vi "Main.vi"(11 "Module Admin":refnum<class "Delacor_lib_QMH_Module Admin.lvclass">) -> ()   [LabVIEW 2025, in "Scripting Server.lvlib"]
doc: "This template is based off of the Queued Message Handler design pattern and the Queued Message Handler project template that ships with LabVIEW.\n\nThe main difference is that the queue is private to this module and communication between modules is performed via Broadcast and Request events.\n\nRequest events are wrapped in public API methods and are handled in the Event Handling Loop (EHL) of this VI. Any module can register for Broadcast events sent by this module. The EHL generates messages based on user interface actions.\n\nThe Message Handling Loop (MHL) processes messages generated by the EHL, or by other messages. The messages are string values, so new messages can be added easily to the Message Cases case structure in the MHL. Each message cluster can also provide an optional value for Message Data, which is a variant that can be converted to whatever message-specific data is required.\n_____\nBased on DQMH Dev Tools: Project Template 7.1.0.1503."
uses:
  Scripting Server.lvlib
  <vilib>/Delacor/Delacor QMH/Libraries/Message Queue_class/Delacor_lib_QMH_Message Queue.lvclass/Delacor_lib_QMH_Message Queue.ctl
  <vilib>/Delacor/Delacor QMH/Libraries/Module Admin_class/Delacor_lib_QMH_Module Admin.lvclass/Delacor_lib_QMH_Module Admin.ctl
  <vilib>/Delacor/Delacor QMH/Libraries/Message Queue_class/Delacor_lib_QMH_Message Queue.lvclass
  Module Data--cluster.ctl
  <vilib>/Utility/miscctls.llb/LVPointTypeDef.ctl
  <vilib>/Delacor/Delacor QMH/Libraries/Message Queue_class/Delacor_lib_QMH_Enqueue Message (Single).vi
  Stop Argument--cluster.ctl
  <vilib>/Delacor/Delacor QMH/Libraries/Module Admin_class/Delacor_lib_QMH_Module Admin.lvclass
  New VI (Reply Payload)--cluster.ctl
  New VI Argument--cluster.ctl
  Add Object Argument--cluster.ctl
  Add Object (Reply Payload)--cluster.ctl
  Connect Objects (Reply Payload)--cluster.ctl
  Connect Objects Argument--cluster.ctl
  Get Object Terminals (Reply Payload)--cluster.ctl
  Get Object Terminals Argument--cluster.ctl
  get vi error list (Reply Payload)--cluster.ctl
  get vi error list Argument--cluster.ctl
  Cleanup VI (Reply Payload)--cluster.ctl
  Cleanup VI Argument--cluster.ctl
  create_control (Reply Payload)--cluster.ctl
  create_control Argument--cluster.ctl
  Run VI (Reply Payload)--cluster.ctl
  Run VI Argument--cluster.ctl
  add_to_selection (Reply Payload)--cluster.ctl
  add_to_selection Argument--cluster.ctl
  clear_selection_list (Reply Payload)--cluster.ctl
  clear_selection_list Argument--cluster.ctl
  remove_from_selection (Reply Payload)--cluster.ctl
  remove_from_selection Argument--cluster.ctl
  enclose_selection (Reply Payload)--cluster.ctl
  enclose_selection Argument--cluster.ctl
  rename_object (Reply Payload)--cluster.ctl
  rename_object Argument--cluster.ctl
  set_value (Reply Payload)--cluster.ctl
  set_value Argument--cluster.ctl
  delete_object (Reply Payload)--cluster.ctl
  delete_object Argument--cluster.ctl
  save_vi (Reply Payload)--cluster.ctl
  save_vi Argument--cluster.ctl
  get_structure_diagram (Reply Payload)--cluster.ctl
  get_structure_diagram Argument--cluster.ctl
  add_subvi (Reply Payload)--cluster.ctl
  add_subvi Argument--cluster.ctl
  connect_to_pane (Reply Payload)--cluster.ctl
  connect_to_pane Argument--cluster.ctl
  get_object_help (Reply Payload)--cluster.ctl
  get_object_help Argument--cluster.ctl
  get_loop_conditional_terminal (Reply Payload)--cluster.ctl
  get_loop_conditional_terminal Argument--cluster.ctl
  show_conditional_terminal (Reply Payload)--cluster.ctl
  show_conditional_terminal Argument--cluster.ctl
  get_loop_iteration_terminal (Reply Payload)--cluster.ctl
  get_loop_iteration_terminal Argument--cluster.ctl
  Config Data.ctl
  Read Config Data Argument--cluster.ctl
  get_allowed_paths (Reply Payload)--cluster.ctl
  get_allowed_paths Argument--cluster.ctl
  create_project (Reply Payload)--cluster.ctl
  create_project Argument--cluster.ctl
  Set Allowed Paths Argument--cluster.ctl
  open_vi (Reply Payload)--cluster.ctl
  open_vi Argument--cluster.ctl
panel:
  in  "Ring 2":i32(ring)=2125 items=[".NET Container"=2125, ".NET Refnum"=3441, "2D Picture"=3508, "3D Picture"=23776, "Absolute Value"=1054, "Accept TLS"=1732, "Access Rights"=1412, "ActiveX Container"=2072, "Add"=1050, "Add (with error terminals)"=3915, "Add Array Elements"=1903, "Add Entropy"=1738, "Add Private Key To TLS Configuration"=1735, "Add Trusted Certificate To TLS Configuration"=1736, "Agitator"=3831, "AllSpoll"=1960, "Always Copy"=2400, "And"=1061, "And Array Elements"=1911, "Append True/False String"=1511, "Application Refnum"=3412, "Array (block diagram constant)"=2070, "Array (classic)"=3300, "Array (modern)"=21608, "Array Interface Control"=23777, "Array Max & Min"=1907, "Array of Strings to Path"=1422, "Array Size"=1809, "Array Subset"=2044, "Array To Cluster"=1168, "Array To Spreadsheet String"=1540, "ArrayMemInfo"=2412, "Assert Structural Type Match"=2416, "Assert Structural Type Mismatch"=2464, "Atmospheric Tank (classic)"=3070, "Atmospheric Tank (modern)"=21751, "Automation Close"=8001, "Automation Open"=8000, "Automation Refnum"=3410, "Avogadro Constant (1/mol)"=23520, "Base 10 Logarithm Of e"=23512, "Bin #1"=3073, "Bin #2"=21755, "Bitpack to Array"=3135, "Bluetooth Close Connection"=9148, "Bluetooth Create Listener"=9151, "Bluetooth Discover"=9152, "Bluetooth Network Connection Refnum"=3468, "Bluetooth Open Connection"=9153, "Bluetooth Read"=9149, "Bluetooth Wait On Listener"=9147, "Bluetooth Write"=9150, "Boolean Array To Number"=1815, "Boolean To (0,1)"=1167, "Build Array"=2041, "Build Cluster Array"=2047, "Build Map"=2463, "Build Matrix"=8500, "Build Path"=1419, "Build Set"=2462, "Build Waveform"=2066, "Bundle"=2049, "Bundle By Name"=2057, "Byte Array To String"=1609, "Byte Array To UTF-8 String"=1651, "Byte Stream File Refnum"=3408, "Call By Reference"=3901, "Call Chain"=1999, "Call Library Function Node"=2062, "Call MATLAB Function"=24210, "Call Parent Class Method"=2354, "CAN Channel (block diagram constant)"=2124, "CAN Channel (classic)"=3340, "CAN Channel (modern)"=21817, "CAN Channel (system)"=21966, "CAN Interface (block diagram constant)"=2123, "CAN Interface (classic)"=3339, "CAN Interface (modern)"=21815, "CAN Interface (system)"=21964, "CAN Task (block diagram constant)"=3471, "CAN Task (classic)"=3470, "CAN Task (modern)"=21789, "CAN Task (system)"=21963, "Cancel Button (modern)"=21739, "Cancel Button (system)"=3131, "Cancel Notification"=9107, "Carriage Return Constant"=23500, "Case Structure"=2001, "Cast Unit Bases"=1079, "Check Valve"=3833, "Checkbox (classic)"=3117, "CheckBox (modern)"=21924, "Checkbox (system)"=3132, "Class Specifier Constant"=2094, "Classic Color Box"=3013, "Classic Color Ramp"=3022, "Classic Horizontal Slide Switch"=3114, "Classic Vertical Slide"=3004, "Clear Fixed-Point Overflow Status"=5562, "Close File"=8052, "Close File (deprecated)"=1405, "Close MATLAB Session"=24209, "Close Python Session"=24207, "Close Reference"=8011, "Close TLS Configuration"=1741, "Close Variable Connection"=23783, "Closure Structure"=2372, "Cluster (classic)"=3400, "Cluster (modern)"=21607, "Cluster Constant"=2071, "Cluster To Array"=1169, "Code Interface Node"=2050, "Coerce To Type"=2402, "Collection Size"=2450, "Color Box Constant"=2120, "Color Box Thin Border"=2905, "Colored Rectangle (broken?)"=3625, "Combo Box (classic)"=3304, "Combo Box (modern)"=21604, "Combo Box (system)"=21917, "Combo Box Constant"=2088, "Complex Conjugate"=1048, "Complex To Polar"=1045, "Complex To Re/Im"=1044, "Compound Arithmetic"=2200, "Compressor"=3832, "Concatenate Strings"=2040, "Conditional Disable Structure"=2064, "Constructor Node"=3904, "Control & Simulation Loop"=2099, "Control Help Window"=1353, "Control Online Help"=1355, "Control Refnum"=3419, "Convert Unit"=2059, "Conveyer"=3827, "Copy"=8053, "Copy (deprecated)"=1416, "Cosecant"=1204, "Cosine"=1201, "Cotangent"=1205, "CPU Information"=24130, "Create Folder"=8055, "Create Network Stream Endpoint"=23793, "Create Network Stream Reader Endpoint"=23811, "Create Network Stream Writer Endpoint"=23810, "Create Stream"=23796, "Create Unique Network Stream Endpoint"=23795, "Create Unique Network Stream Reader Endpoint"=23807, "Create Unique Network Stream Writer Endpoint"=23806, "Create User Event"=2073, "Current Processor ID"=24131, "Current VI's Menubar"=9000, "Current VI's Path"=1426, "DAQmx Analog Trigger Source (block diagram constant)"=2119, "DAQmx Analog Trigger Source (classic)"=3336, "DAQmx Analog Trigger Source (modern)"=21774, "DAQmx Analog Trigger Source (system)"=21951, "DAQmx Device Name (block diagram constant)"=2093, "DAQmx Device Name (classic)"=3318, "DAQmx Device Name (modern)"=21773, "DAQmx Device Name (system)"=21950, "DAQmx Global Channel (block diagram constant)"=3430, "DAQmx Global Channel (classic)"=3443, "DAQmx Global Channel (modern)"=21770, "DAQmx Global Channel (system)"=21957, "DAQmx Physical Channel (block diagram constant)"=2118, "DAQmx Physical Channel (classic)"=3335, "DAQmx Physical Channel (modern)"=21777, "DAQmx Physical Channel (system)"=21954, "DAQmx Scale Name (block diagram constant)"=2116, "DAQmx Scale Name (classic)"=3317, "DAQmx Scale Name (modern)"=21775, "DAQmx Scale Name (system)"=21952, "DAQmx Switch (block diagram constant)"=2121, "DAQmx Switch (classic)"=3337, "DAQmx Switch (modern)"=21776, "DAQmx Switch (system)"=21953, "DAQmx Task Name (block diagram constant)"=3434, "DAQmx Task Name (classic)"=3442, "DAQmx Task Name (modern)"=21778, "DAQmx Task Name (system)"=21959, "DAQmx Terminal (block diagram constant)"=2117, "DAQmx Terminal (classic)"=3319, "DAQmx Terminal (modern)"=21781, "DAQmx Terminal (system)"=21955, "Data Cache Size"=24132, "Data Log File Refnum"=3402, "Data Value Reference"=3476, "Data Value Reference Constant"=24134, "DataSocket Close"=1085, "DataSocket Open"=1084, "DataSocket Read"=1086, "DataSocket Refnum"=3417, "DataSocket Write"=1087, "Date/Time To Seconds"=1308, "Decimal Digit?"=1119, "Decimal String To Number"=1184, "Decimate 1D Array"=2046, "DecomposeLockDataValRef"=2406, "DecomposeVariant"=2404, "Decrement"=1058, "Default Directory"=1427, "Delete"=8056, "Delete (deprecated)"=1417, "Delete Data Value Reference"=2409, "Delete From Array"=3912, "Delete Menu Items"=9004, "Delete Variant Attribute"=8206, "Delete Waveform Attribute"=8209, "Deny Access"=8057, "Dequeue Element"=9113, "Destroy Stream Endpoint"=23794, "Destroy User Event"=2075, "DevClear"=1961, "DevClearList"=1962, "Device Control/Status"=1433, "Device Refnum"=3405, "Diagram Disable Structure"=2054, "Dial (classic)"=3050, "Dial (modern)"=21732, "Digital Data (classic)"=3210, "Digital Data (modern)"=21216, "Digital Waveform Graph (classic)"=3511, "Digital Waveform Graph (modern)"=21718, "Direct Variable Read"=23785, "Direct Variable Write"=23788, "Divide"=1053, "Divide (with error terminals)"=3918, "Dlg Horiz Scrollbar"=21905, "Dlg Mac Group Box"=32514, "Dlg Numeric #1"=2100, "Dlg Numeric #2"=3006, "Dlg String"=2110, "Dlg Vert Scrollbar"=21906, "Down Arrow"=3824, "Down Bow Valve (flat)"=3707, "Down Bow Valve (outline)"=3807, "Down Bow Valve (shaded)"=21767, "Down Rect Valve (flat)"=3706, "Down Rect Valve (outline)"=3806, "Down Rect Valve (shaded)"=21766, "Down Tee (flat)"=3818, "Down Tee (shaded)"=3718, "Dynamic FPGA Interface Cast"=5690, "Eased Corner Rectangle"=32513, "Element of Set?"=2454, "Elementary Charge (C)"=23517, "Empty Array?"=23063, "Empty Collection?"=2451, "Empty Path Constant"=23523, "Empty String Constant"=23503, "Empty String/Path?"=1112, "Enable Menu Tracking"=9002, "EnableLocal"=1963, "EnableRemote"=1964, "End of Line Constant"=23525, "Enqueue Element"=9111, "Enqueue Element At Opposite End"=9129, "Enum (classic)"=3023, "Enum (modern)"=21605, "Enum (system)"=3062, "Enum Constant"=2090, "EOF"=1410, "Equal To 0?"=1113, "Equal?"=1102, "Error Ring Constant"=2039, "Event Callback Refnum"=3435, "Event Data Node"=2102, "Event Structure"=2052, "Exchanger"=3828, "Exclusive Or"=1063, "Exponential"=1211, "Exponential (Arg) -1"=1222, "Expression Node"=2201, "False Constant"=2006, "Feedback Node"=2353, "FieldPoint IO Point (block diagram constant)"=3440, "FieldPoint IO Point (classic)"=3439, "FieldPoint IO Point (modern)"=21784, "FIFO Refnum"=3474, "File Dialog"=8058, "File Dialog (deprecated)"=8081, "File Path Control (classic)"=3203, "File Path Control (modern)"=21730, "File Path Control (system)"=21922, "File Path Indicator (classic)"=3204, "File Path Indicator (modern)"=21731, "File/Directory Info"=8082, "File/Directory Info (deprecated)"=1413, "FindLstn"=1965, "FindRQS"=1966, "First Call?"=1083, "Fixed-Point Overflow?"=5565, "Fixed-Point to Integer Cast"=5566, "Flat Box"=3602, "Flat Circle"=3605, "Flat Down Triangle"=3623, "Flat Frame"=3608, "Flat Left Triangle"=3620, "Flat Right Triangle"=3621, "Flat Round Button"=3102, "Flat Rounded Box"=3611, "Flat Sequence Structure"=2069, "Flat Square Button"=3103, "Flat Up Triangle"=3622, "Flatten To JSON"=24201, "Flatten To String"=1164, "Flatten To XML"=8402, "Flattened String To Variant"=8202, "Floating Point Equal?"=23064, "Flush Event Queue"=2135, "Flush File"=8059, "Flush File (deprecated)"=1406, "Flush Queue"=9114, "Flush Stream"=23808, "For Loop"=2002, "Fork"=2194, "Format Date/Time String"=8100, "Format Into File"=2083, "Format Into String"=2081, "Format Value"=1512, "Formula Node"=2004, "FPGA Refnum to Session"=2322, "Fract/Exp String To Number"=1187, "Framed Color Box (classic)"=3008, "Framed Color Box (modern)"=21019, "Free Label"=2321, "Furnace"=3829, "Gauge (classic)"=3040, "Gauge (modern)"=21009, "Gauge for Simon"=32600, "Generate Front Panel Activity"=1329, "Generate Occurrence"=1700, "Generate User Event"=2074, "Generate User-Defined Trace Event"=2250, "Get Control Values by Index"=24204, "Get Datalog Position"=8061, "Get Date/Time In Seconds"=1303, "Get Date/Time String"=1600, "Get Drag Drop Data"=9154, "Get File Position"=8062, "Get File Size"=8063, "Get Fixed-Point Components"=11163, "Get Help Window Status"=1354, "Get Matrix Diagonal"=8501, "Get Matrix Elements"=8502, "Get Menu Item Info"=9005, "Get Menu Selection"=9001, "Get Menu Short Cut Info"=9007, "Get Notifier Status"=9103, "Get Number of Records"=8064, "Get Permissions"=8065, "Get Queue Status"=9110, "Get Submatrix"=8503, "Get Type and Creator"=8066, "Get Variant Attribute"=8205, "Get Volume Info"=8067, "Get Waveform Attribute"=8208, "Get Waveform Components"=2067, "Global Variable"=2060, "GPIB Clear"=1954, "GPIB Initialization"=1957, "GPIB Misc"=1956, "GPIB Read"=1951, "GPIB Serial Poll"=1955, "GPIB Status"=1959, "GPIB Trigger"=1953, "GPIB Wait"=1958, "GPIB Write"=1950, "Gravitational Constant (N m2/kg2)"=23519, "Greater Or Equal To 0?"=1114, "Greater Or Equal?"=1103, "Greater Than 0?"=1117, "Greater?"=1110, "Handle Peek"=1604, "Handle Poke"=1605, "Hex Digit?"=1123, "Hexadecimal String To Number"=1185, "Hopper #1"=21754, "Hopper #2"=3072, "Horiz Line"=3821, "Horiz Pipe (flat)"=3810, "Horiz Pipe (shaded)"=3710, "Horizontal Button Box"=3636, "Horizontal Fill Slide (classic)"=3012, "Horizontal Fill Slide (modern)"=21100, "Horizontal Gradient Oval"=32502, "Horizontal Gradient Rectangle"=32504, "Horizontal Gradient Rounded Rectangle"=32507, "Horizontal Graduated Bar"=21106, "Horizontal Pointer Slide (classic)"=3011, "Horizontal Pointer Slide (modern)"=21101, "Horizontal Pointer Slide (system)"=21902, "Horizontal Progress Bar (modern)"=21102, "Horizontal Progress Bar (system)"=21910, "Horizontal Scrollbar"=21110, "Horizontal Slide (classic)"=3010, "Horizontal Slide (system)"=21904, "Horizontal Smooth Box"=3633, "Horizontal Splitter Bar"=21861, "Horizontal Splitter Bar (Classic)"=21863, "Horizontal Splitter Bar (NXG Style)"=21867, "Horizontal Splitter Bar (System)"=21865, "Horizontal Switch"=3108, "Horizontal Tank"=3071, "Horizontal Toggle Switch (classic)"=3110, "Horizontal Toggle Switch (modern)"=21700, "Hyperbolic Cosecant"=23053, "Hyperbolic Cosine"=1215, "Hyperbolic Cotangent"=23055, "Hyperbolic Secant"=23054, "Hyperbolic Sine"=1214, "Hyperbolic Tangent"=1216, "IMAQ Session"=3415, "Implies"=1080, "In Place Element Structure"=2360, "In Range and Coerce"=1127, "Include Fixed-Point Overflow Status"=5564, "Increment"=1057, "Index & Bundle Cluster Array"=2056, "Index Array"=2042, "Index String Array"=1531, "Initialize Array"=2053, "Inline C Node"=2104, "Insert Into Array"=3911, "Insert Into Map"=2456, "Insert Into Set"=2452, "Insert Menu Items"=9003, "Integer to Fixed-Point Cast"=5567, "Intensity Chart (classic)"=3509, "Intensity Chart (modern)"=21719, "Intensity Graph (classic)"=3510, "Intensity Graph (modern)"=21720, "Interleave 1D Arrays"=2045, "Interpolate 1D Array"=1905, "Inverse Cosecant"=23050, "Inverse Cosine"=1207, "Inverse Cotangent"=23052, "Inverse Hyperbolic Cosecant"=23056, "Inverse Hyperbolic Cosine"=1218, "Inverse Hyperbolic Cotangent"=23058, "Inverse Hyperbolic Secant"=23057, "Inverse Hyperbolic Sine"=1217, "Inverse Hyperbolic Tangent"=1219, "Inverse Secant"=23051, "Inverse Sine"=1206, "Inverse Tangent"=1208, "Inverse Tangent (2 Input)"=1228, "Invoke Node"=3900, "IP To String"=1710, "IrDA Close Connection"=9144, "IrDA Create Listener"=9140, "IrDA Discover"=9141, "IrDA Network Connection Refnum"=3450, "IrDA Open Connection"=9142, "IrDA Read"=9145, "IrDA Wait On Listener"=9143, "IrDA Write"=9146, "IsDebuggingActive"=2403, "IVI Delete Session"=8103, "IVI Logical Name (block diagram constant)"=3420, "IVI Logical Name (classic)"=3414, "IVI Logical Name (modern)"=21736, "IVI New Session"=8102, "Join"=2195, "Join Numbers"=1171, "Junction"=2197, "Knob (classic)"=3005, "Knob (modern)"=21000, "Label (modern)"=21960, "Label (system)"=21961, "Labeled Oblong Button"=3125, "Labeled Rectangular Button"=3124, "Labeled Round Button"=3122, "Labeled Square Button"=3123, "LabVIEW Object"=3457, "Leak Variant Value Reference"=2410, "LED Button"=3116, "Left Arrow"=3826, "Left Bow Valve (flat)"=3701, "Left Bow Valve (outline)"=3801, "Left Bow Valve (shaded)"=21761, "Left Down Elbow (flat)"=3811, "Left Down Elbow (shaded)"=3711, "Left Pump (flat)"=3813, "Left Pump (shaded)"=3713, "Left Rect Valve (flat)"=3700, "Left Rect Valve (outline)"=3800, "Left Rect Valve (shaded)"=21760, "Left Tee (flat)"=3809, "Left Tee (shaded)"=3709, "Left Up Elbow (flat)"=3808, "Left Up Elbow (shaded)"=3708, "Less Or Equal To 0?"=1115, "Less Or Equal?"=1104, "Less Than 0?"=1118, "Less?"=1111, "Lexical Class"=1126, "Line (chiseled, system)"=3632, "Line (chiseled, thick)"=3630, "Line (chiseled, thin)"=3627, "Line (thick)"=3629, "Line (thin)"=3626, "Line Feed Constant"=23501, "Line with Arrow (thick)"=3631, "Line with Arrow (thin)"=3628, "List Directory"=1418, "List Folder"=8083, "Listbox (classic)"=21806, "Listbox (modern)"=21792, "Listbox (system)"=21805, "Listbox Symbol Ring Constant"=2038, "Load Certificates Into Memory"=1734, "Load Private Key Into Memory"=1733, "Local Variable"=2061, "Lock Range"=1411, "Logarithm Base 10"=1210, "Logarithm Base 2"=1225, "Logarithm Base X"=1224, "Logical Shift"=1081, "Look In Map"=2458, "Lookup Channel Probe"=9155, "Lossy Enqueue Element"=9130, "Lowered Box (thick)"=3635, "Lowered Rounded Box"=3638, "Machine Epsilon"=23528, "Make TLS Configuration Immutable"=1737, "MakeAddr"=1967, "Mantissa & Exponent"=1150, "Map"=3488, "Map Constant"=2461, "Match First String"=1532, "Match Pattern"=1535, "Match True/False String"=1533, "MathScript Call By Reference"=3906, "MathScript Node"=2357, "MATLAB script"=9020, "MATLAB Session Refnum"=3490, "Matrix Size"=8507, "Max & Min"=1108, "Menu Refnum"=3413, "Menu Ring (classic)"=3018, "Menu Ring (modern)"=21600, "Menu-Popup Ring"=3017, "Merge Errors"=2147, "Merge Signals"=2350, "Meter (classic)"=3030, "Meter (modern)"=21008, "Mixed Checkbox (system)"=21333, "Mixed Signal Graph"=21721, "Molar Gas Constant (J/(mol K))"=23522, "Motion Resource (block diagram constant)"=3449, "Motion Resource (classic)"=3448, "Motion Resource (modern)"=21787, "Motor (flat)"=3820, "Motor (shaded)"=3720, "Move"=8068, "Move (deprecated)"=1415, "Multi-Segment Pipe"=23780, "Multicolumn Listbox (classic)"=21799, "Multicolumn Listbox (modern)"=21791, "Multicolumn Listbox (system)"=21798, "Multiply"=1052, "Multiply (with error terminals)"=3917, "Multiply Array Elements"=1904, "Multirate Structure"=2199, "Natural Logarithm"=1209, "Natural Logarithm (Arg +1)"=1221, "Natural Logarithm Base"=23510, "Natural Logarithm Of 10"=23513, "Natural Logarithm Of 2"=23514, "Natural Logarithm Of Pi"=23508, "Negate"=1069, "Negative Infinity"=23509, "New Data Value Reference"=2408, "New Directory"=1402, "New File"=1404, "New TLS Configuration"=1730, "New VI"=8014, "New VI Object"=8015, "Not"=1064, "Not A Number/Path/Refnum?"=1128, "Not A Path Constant"=23524, "Not a Refnum Constant"=23526, "Not a Shared Variable"=23527, "Not And"=1071, "Not Equal To 0?"=1116, "Not Equal?"=1105, "Not Exclusive Or"=1073, "Not Or"=1072, "Notifier Refnum"=3423, "Number of Cache Levels"=24133, "Number To Boolean Array"=1814, "Number To Decimal String"=1180, "Number To Engineering String"=1183, "Number To Exponential String"=1505, "Number To Fractional String"=1506, "Number To Hexadecimal String"=1181, "Number To Octal String"=1182, "Numeric Constant"=2005, "Numeric Control (classic)"=3000, "Numeric Control (modern)"=21003, "Numeric Control (system)"=21919, "Numeric Indicator (classic)"=3001, "Numeric Indicator (modern)"=21004, "Obtain Notifier"=9101, "Obtain Queue"=9108, "Occurrence Refnum"=3406, "Octal Digit?"=1129, "Octal String To Number"=1186, "OK Button (modern)"=21738, "OK Button (system)"=3130, "Old VISA Open"=1921, "OLE Variant"=3150, "One Button Dialog"=1340, "Open and Verify Variable Connection"=23790, "Open Application Reference"=8012, "Open Device"=1430, "Open Dynamic Bitfile Reference"=5691, "Open File"=1403, "Open MATLAB Session"=24208, "Open Python Session"=24206, "Open Tank (flat classic)"=21752, "Open Tank (shaded classic)"=3074, "Open Variable Connection"=23779, "Open Variable Connection in Background"=23791, "Open VI Object Reference"=8013, "Open VI Reference"=8010, "Open/Create/Replace Datalog"=8054, "Open/Create/Replace File"=8050, "Or"=1062, "Or Array Elements"=1910, "Oval with Shadow"=32509, "Package Matrix"=23001, "PassControl"=1968, "Path Constant"=2009, "Path to Array of Strings"=1423, "Path To String"=1077, "Path Type"=1421, "Pi"=23504, "Pi Divided By 2"=23506, "Pi Multiplied By 2"=23505, "Pick Line"=1510, "Pict Ring (classic)"=3015, "Pict Ring (modern)"=21602, "Pict Ring (system)"=21925, "PixMap"=3505, "PixMap (warning: dangerous)"=3507, "Planck's Constant (J/Hz)"=23516, "Platform Flat Square Button"=3134, "Plug-In Control"=21820, "Polar To Complex"=1047, "Polar To Re/Im"=23061, "Positive Infinity"=23515, "Power Of 10"=1212, "Power Of 2"=1223, "Power Of X"=1213, "PPoll"=1969, "PPollConfig"=1970, "PPollUnconfig"=1971, "Preallocated Read from Binary File"=24135, "Preserve Run-Time Class"=8018, "Pressure Tank (flat)"=3075, "Pressure Tank (shaded)"=21753, "Preview Queue Element"=9112, "Printable?"=1124, "Property Node"=1920, "Pulldown Menu Ring"=3061, "Push Button"=21001, "Python Node"=24205, "Python Session Refnum"=3486, "Queue Refnum"=3424, "Quit LabVIEW"=1352, "Quotient & Remainder"=1056, "Race Structure"=2371, "Radio Button (system)"=3133, "Radio Buttons (classic)"=22003, "Radio Buttons (modern)"=22001, "Radio Buttons (system)"=22002, "Raised Box (classic)"=3600, "Raised Box (modern)"=3637, "Raised Circle"=3603, "Raised Down Triangle"=3615, "Raised Frame"=3606, "Raised Left Triangle"=3612, "Raised Right Triangle"=3613, "Raised Rounded Box"=3609, "Raised Up Triangle"=3614, "Random Number (0-1)"=1070, "RcvRespMsg"=1972, "Re-accept TLS"=1739, "Re/Im To Complex"=1046, "Re/Im To Polar"=23060, "Read Datalog"=8069, "Read Device"=1432, "Read File"=1407, "Read from Binary File"=8051, "Read from Text File"=8070, "Read Map Max & Min Keys"=2459, "Read Multiple Elements from Stream"=23803, "Read Set Max & Min"=2455, "Read Single Element from Stream"=23797, "Read Variable"=23781, "Read Variable with Timeout"=23786, "ReadStatus"=1973, "Receive"=1974, "ReceiveSetup"=1975, "Recessed Box"=3601, "Recessed Circle"=3604, "Recessed Down Triangle"=3619, "Recessed Frame (modern)"=3607, "Recessed Frame (system)"=3624, "Recessed Left Triangle"=3616, "Recessed Menu Ring"=3019, "Recessed Right Triangle"=3617, "Recessed Rounded Box"=3610, "Recessed Up Triangle"=3618, "Reciprocal"=1059, "Reciprocal Of e"=23511, "Reciprocal Of Pi"=23507, "RecomposeUnlockDataValRef (warning: dangerous)"=2407, "RecomposeVariant (warning: dangerous)"=2405, "Rectangular Stop Button"=3128, "Refnum to Path"=1424, "Refnum to Session"=2306, "Region"=2196, "Register Event Callback"=2078, "Register For Events"=2065, "Register Session"=2319, "Release Notifier"=9102, "Release Queue"=9109, "Remove Fixed-Point Overflow Status"=5563, "Remove From Map"=2457, "Remove From Set"=2453, "Replace Array Subset"=3910, "Replace Substring"=3913, "Request Deallocation"=1610, "ResetSys"=1976, "Reshape Array"=2055, "Resize Matrix"=8508, "Resource Index"=1088, "Reverse 1D Array"=1900, "Reverse String"=1537, "Right Arrow"=3825, "Right Bow Valve (flat)"=3705, "Right Bow Valve (outline)"=3805, "Right Bow Valve (shaded)"=21765, "Right Down Elbow (flat)"=3817, "Right Down Elbow (shaded)"=3717, "Right Pump (flat)"=3819, "Right Pump (shaded)"=3719, "Right Rect Valve (flat)"=3704, "Right Rect Valve (outline)"=3804, "Right Rect Valve (shaded)"=21764, "Right Tee (flat)"=3815, "Right Tee (shaded)"=3715, "Right Up Elbow (flat)"=3814, "Right Up Elbow (shaded)"=3714, "Rocker"=21002, "Rotary Feeder"=3830, "Rotate"=1082, "Rotate 1D Array"=1906, "Rotate Left With Carry"=1606, "Rotate Right With Carry"=1607, "Rotate String"=1536, "Round Button"=3100, "Round LED (classic)"=3120, "Round LED (modern)"=21012, "Round Light"=3104, "Round Push Button"=3118, "Round Push Button (profile)"=3112, "Round Radio Button"=3106, "Round Stop Button"=3127, "Round To Nearest"=1055, "Round Toward +Infinity"=1076, "Round Toward -Infinity"=1075, "Rounded Rectangle with Shadow"=32508, "RT FIFO Create"=24000, "RT FIFO Delete"=24003, "RT FIFO Read"=24001, "RT FIFO Write"=24002, "Rydberg Constant (1/m)"=23521, "Scale By Power Of 2"=1074, "Scan From File"=2082, "Scan From String"=2080, "Scan String For Tokens"=8101, "Scan Value"=1534, "Scanned Variable Read"=23784, "Scanned Variable Write"=23787, "Search 1D Array"=1901, "Search and Replace String"=3914, "Search Variable Container"=23802, "Search/Split String"=1538, "Secant"=1203, "Seconds To Date/Time"=1309, "Seek"=1409, "Select"=1516, "Send"=1977, "Send Notification"=9104, "SendCmds"=1978, "SendDataBytes"=1979, "SendIFC"=1980, "SendList"=1981, "SendLLO"=1982, "SendSetup"=1983, "Session to Refnum"=2307, "Set"=3487, "Set Constant"=2460, "Set Control Values by Index"=24203, "Set Datalog Position"=8072, "Set File Position"=8073, "Set File Size"=8074, "Set Matrix Diagonal"=8504, "Set Matrix Elements"=8505, "Set Menu Item Info"=9006, "Set Number of Records"=8075, "Set Occurrence"=1702, "Set Permissions"=8076, "Set Submatrix"=8506, "Set Type and Creator"=8077, "Set Variant Attribute"=8204, "Set Waveform Attribute"=8207, "SetRWLS"=1984, "SetTimeOut"=1985, "Shared Variable"=23778, "Shared Variable Constant"=3473, "Shared Variable Control (classic)"=3472, "Shared Variable Control (modern)"=21814, "Shared Variable to String"=1831, "Sign"=1049, "Simple Horizontal Slide"=3003, "Simple Numeric"=2900, "Simple String"=2115, "Simple Vertical Slide"=3002, "Sinc"=1227, "Sine"=1200, "Sine & Cosine"=1220, "Size Handle"=1603, "Slide Switch"=21011, "Smoothed Oval"=32500, "Smoothed Rounded Rectangle"=32505, "Sort 1D Array"=1120, "Sort Array of String"=23065, "Speed Of Light In Vacuum (m/sec)"=23518, "Spin Control (system)"=21900, "Split 1D Array"=1908, "Split Button"=21020, "Split Number"=1170, "Split Signals"=2351, "Spreadsheet String To Array"=1539, "Square"=23059, "Square Button"=3101, "Square LED (classic)"=3121, "Square LED (modern)"=21013, "Square Light"=3105, "Square Push Button"=3119, "Square Push Button (profile)"=3113, "Square Radio Button"=3107, "Square Root"=1060, "Stacked Sequence Structure"=2000, "Start TLS"=1731, "State"=2198, "State Diagram"=2051, "Static VI Reference"=2084, "Stop"=1350, "Stop Button"=21230, "String Constant"=2007, "String Control (classic)"=3200, "String Control (modern)"=21701, "String Control (system)"=21920, "String Indicator (classic)"=3201, "String Indicator (modern)"=21702, "String Length"=1502, "String Subset"=1503, "String To Byte Array"=1608, "String To IP"=1711, "String To Path"=1078, "String to Shared Variable"=1830, "Strip Path"=1420, "SubPanel"=21810, "SubPanel (Classic)"=21811, "SubPanel (NXG Style)"=21824, "SubPanel (System)"=21823, "Subtract"=1051, "Subtract (with error terminals)"=3916, "Swap Bytes"=1162, "Swap Values"=2401, "Swap Vector Element"=1912, "Swap Words"=1163, "Tab Constant"=23502, "Tab Control (classic)"=3330, "Tab Control (modern)"=3332, "Tab Control (NXG Style)"=32700, "Tab Control (system)"=3331, "Table (classic)"=21796, "Table (modern)"=21790, "Table (system)"=21797, "Tag Attribute Ring"=2063, "Tangent"=1202, "Tank (classic)"=3020, "Tank (modern)"=21006, "Target Structure"=2370, "TCP Close Connection"=1713, "TCP Create Listener"=1717, "TCP Flattened Read"=1718, "TCP Flattened Write"=1719, "TCP Flex Read"=1720, "TCP Flex Write"=1721, "TCP Network Connection Refnum"=3407, "TCP Open Connection"=1715, "TCP Read"=1716, "TCP Wait On Listener"=1712, "TCP Write"=1714, "TDMS Advanced Asynchronous Read (Data Ref)"=2151, "TDMS Advanced Asynchronous Write (Data Ref)"=2150, "TDMS Close"=24113, "TDMS Configure Asynchronous Reads (Data Ref)"=2153, "TDMS Configure Asynchronous Writes (Data Ref)"=2152, "TDMS Defragment"=24119, "TDMS Delete Data"=2159, "TDMS File"=3477, "TDMS Flush"=24117, "TDMS Get Asynchronous Read Status (Data Ref)"=2155, "TDMS Get Asynchronous Write Status (Data Ref)"=2154, "TDMS Get Properties"=24115, "TDMS In Memory Close"=2157, "TDMS In Memory Open"=2156, "TDMS In Memory Read Bytes"=2158, "TDMS List Contents"=24116, "TDMS Open"=24112, "TDMS Read"=24111, "TDMS Refnum To File ID"=24120, "TDMS Set Properties"=24114, "TDMS Write"=24110, "TDMS Write IP"=24118, "Temporary Directory"=1435, "TestSRQ"=1986, "TestSys"=1987, "Text & Pict Ring (classic)"=3016, "Text & Pict Ring (modern)"=21603, "Text Button"=21015, "Text Ring (block diagram constant)"=2008, "Text Ring (classic)"=3014, "Text Ring (modern)"=21601, "Text Ring (system)"=3060, "Text to UTF-8"=23066, "Thermometer (classic)"=3021, "Thermometer (modern)"=21007, "Threshold 1D Array"=1909, "Tick Count (ms)"=1300, "Time Stamp (block diagram constant)"=2068, "Time Stamp Control (classic)"=5555, "Time Stamp Control (modern)"=21913, "Time Stamp Control (system)"=21967, "Time Stamp Indicator (classic)"=5556, "Time Stamp Indicator (modern)"=21914, "Timed Loop"=5570, "Timed Sequence"=5573, "TLS configuration"=3489, "TLS Connection?"=1740, "To Byte Integer"=1140, "To Double Precision Complex"=1152, "To Double Precision Float"=1147, "To Extended Precision Complex"=1154, "To Extended Precision Float"=1149, "To Fixed-Point"=5561, "To Long Integer"=1142, "To Lower Case"=1189, "To More Generic Class"=8017, "To More Specific Class"=8016, "To OLE Variant"=8002, "To Probe String"=2413, "To Quad Integer"=1155, "To Single Precision Complex"=1151, "To Single Precision Float"=1146, "To Time Stamp"=5560, "To Unsigned Byte Integer"=1143, "To Unsigned Long Integer"=1145, "To Unsigned Quad Integer"=1156, "To Unsigned Word Integer"=1144, "To Upper Case"=1188, "To Variant"=8201, "To Word Integer"=1141, "Traditional DAQ Channel (block diagram constant)"=2085, "Traditional DAQ Channel (classic)"=3320, "Traditional DAQ Channel (modern)"=21733, "Transpose 1D Array"=23068, "Transpose 2D Array"=1902, "Transpose Matrix"=8509, "Tree (classic)"=21819, "Tree (modern)"=21793, "Tree (system)"=21794, "Trigger"=1988, "TriggerList"=1989, "Two Button Dialog"=1341, "Type and Creator"=1434, "Type Cast"=1166, "Type Error"=2415, "Type Must Be Array"=2417, "Type Must Be Cluster"=2418, "Type Of"=2414, "Type Specialization Structure"=2373, "UDP Close"=1726, "UDP Multicast Open"=1727, "UDP Network Connection Refnum"=3418, "UDP Open"=1723, "UDP Read"=1724, "UDP Write"=1725, "Unbitpack from Array"=3136, "Unbundle"=2048, "Unbundle By Name"=2058, "Unflatten From JSON"=24202, "Unflatten From String"=1165, "Unflatten From XML"=8401, "Unleak Variant Value Reference"=2411, "Unpackage Matrix"=23000, "Unregister For Events"=2076, "Unregister Session"=2320, "Up Arrow"=3823, "Up Bow Valve (flat)"=3703, "Up Bow Valve (outline)"=3803, "Up Bow Valve (shaded)"=21763, "Up Rect Valve (flat)"=3702, "Up Rect Valve (outline)"=21762, "Up Rect Valve (shaded)"=3802, "Up Tee (flat)"=3812, "Up Tee (shaded)"=3712, "User Defined Refnum"=3428, "User Defined Refnum Tag (block diagram constant)"=3426, "User Defined Refnum Tag (classic)"=3429, "User Defined Refnum Tag (modern)"=21745, "User Defined Refnum Tag Flatten (classic)"=3454, "User Defined Refnum Tag Flatten (modern)"=21747, "User Defined Tag (block diagram constant)"=2114, "User Defined Tag (classic)"=3329, "User Defined Tag (modern)"=21749, "User Item"=3506, "UTF-8 String To Byte Array"=1650, "UTF-8 to Text"=23067, "Variable Class Specifier Constant"=2106, "Variable Name Constant"=3478, "Variant"=3310, "Variant To Data"=8003, "Variant To Flattened String"=8203, "Vert Line"=3822, "Vert Pipe (flat)"=3816, "Vert Pipe (shaded)"=3716, "Vert Rocker"=21740, "Vertical Fill Slide (classic)"=3009, "Vertical Fill Slide (modern)"=21014, "Vertical Gradient Oval"=32501, "Vertical Gradient Rectangle"=32503, "Vertical Gradient Rounded Rectangle"=32506, "Vertical Graduated Bar"=21107, "Vertical Pointer Slide (classic)"=3007, "Vertical Pointer Slide (modern)"=21017, "Vertical Pointer Slide (system)"=21901, "Vertical Progress Bar (modern)"=21104, "Vertical Progress Bar (system)"=21909, "Vertical Scrollbar"=21111, "Vertical Slide (system)"=21903, "Vertical Slide Switch (classic)"=3115, "Vertical Slide Switch (modern)"=21741, "Vertical Smooth Box"=3634, "Vertical Splitter Bar"=21860, "Vertical Splitter Bar (Classic)"=21862, "Vertical Splitter Bar (NXG Style)"=21866, "Vertical Splitter Bar (System)"=21864, "Vertical Switch"=3109, "Vertical Toggle Switch (classic)"=3111, "Vertical Toggle Switch (modern)"=21005, "VI Library"=1425, "VI Refnum"=3422, "VI Server Reference"=2091, "VISA Assert Interrupt Signal"=2309, "VISA Assert Trigger"=1929, "VISA Assert Utility Signal"=2310, "VISA Clear"=1927, "VISA Close"=1922, "VISA Disable Event"=1940, "VISA Discard Events"=1941, "VISA Enable Event"=1942, "VISA Find Resource"=1923, "VISA Flush I/O Buffer"=2302, "VISA GPIB Command"=2315, "VISA GPIB Control ATN"=2316, "VISA GPIB Control REN"=2304, "VISA GPIB Pass Control"=2317, "VISA GPIB Send IFC"=2318, "VISA In 16"=1930, "VISA In 32"=1944, "VISA In 64"=2140, "VISA In 8"=1936, "VISA Lock"=1993, "VISA Map Address"=1932, "VISA Map Trigger"=2311, "VISA Memory Allocation"=1997, "VISA Memory Allocation Ex"=2146, "VISA Memory Free"=1998, "VISA Move"=2303, "VISA Move In 16"=1948, "VISA Move In 32"=1991, "VISA Move In 64"=2144, "VISA Move In 8"=1946, "VISA Move Out 16"=1949, "VISA Move Out 32"=1992, "VISA Move Out 64"=2145, "VISA Move Out 8"=1947, "VISA Open"=2308, "VISA Out 16"=1931, "VISA Out 32"=1945, "VISA Out 64"=2141, "VISA Out 8"=1937, "VISA Peek 16"=1934, "VISA Peek 32"=1995, "VISA Peek 64"=2142, "VISA Peek 8"=1938, "VISA Poke 16"=1935, "VISA Poke 32"=1996, "VISA Poke 64"=2143, "VISA Poke 8"=1939, "VISA Read"=1925, "VISA Read STB"=1928, "VISA Read To File"=2313, "VISA Refnum to Session"=2300, "VISA Resource Name"=3421, "VISA resource name (classic)"=3409, "VISA resource name (modern)"=21737, "VISA Set I/O Buffer Size"=2301, "VISA Status Description"=1924, "VISA Unlock"=1994, "VISA Unmap Address"=1933, "VISA Unmap Trigger"=2312, "VISA USB Control In"=2086, "VISA USB Control Out"=2087, "VISA VXI Cmd or Query"=2305, "VISA Wait on Event"=1943, "VISA Write"=1926, "VISA Write From File"=2314, "Volume Info"=1414, "Wait (ms)"=1302, "Wait For Activity"=1722, "Wait For Front Panel Activity"=1328, "Wait for GPIB RQS"=1952, "Wait on Notification"=9105, "Wait on Notification from Multiple"=9106, "Wait on Notification from Multiple with Notifier History"=9132, "Wait on Notification with Notifier History"=9131, "Wait on Occurrence"=1701, "Wait Until Next ms Multiple"=1327, "WaitSRQ"=1990, "Waveform Chart"=21010, "Waveform Chart (classic)"=3501, "Waveform Chart (modern)"=21717, "Waveform Graph (classic)"=3504, "Waveform Graph (modern)"=21703, "While Loop #1"=2003, "While Loop #2"=2352, "White Space?"=1125, "Write Datalog"=8079, "Write Device"=1431, "Write File"=1408, "Write Multiple Elements to Stream"=23804, "Write Single Element to Stream"=23798, "Write to Binary File"=8078, "Write to Text File"=8080, "Write Variable"=23782, "Write Variable with Timeout"=23789, "XY Graph (classic)"=3500, "XY Graph (modern)"=21716, "Y-th Root of X"=23062]
  out "error out":errorcluster
  out "Status":string
  in  "Simulate MHL Error":bool
  in  "Simulate EHL Error":bool
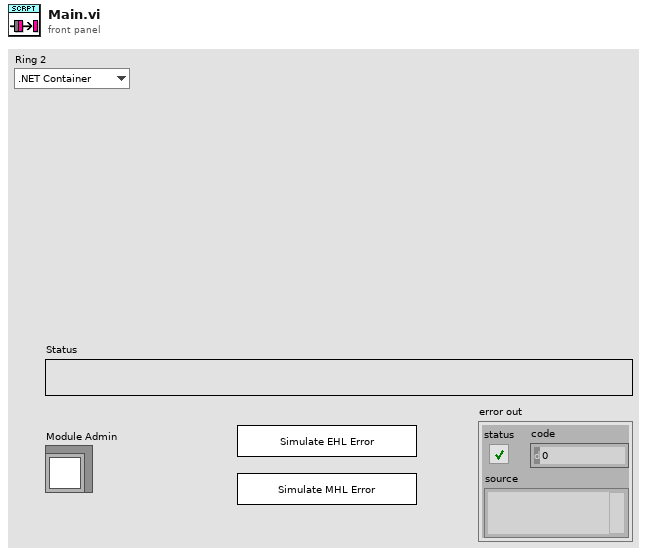
[diagram p1: front panel]
types:
  T1 = typedef "Scripting Server.lvlib/Request Events--cluster.ctl" = cluster{"Stop Module":refnum<user-event>, "Show Panel":refnum<user-event>, "Hide Panel":refnum<user-event>, "Get Module Execution Status":refnum<user-event>, "Show Diagram":refnum<user-event>, "New VI":refnum<user-event>, "Add Object":refnum<user-event>, "Connect Objects":refnum<user-event>, "Get Object Terminals":refnum<user-event>, "get vi error list":refnum<user-event>, "Cleanup VI":refnum<user-event>, "create_control":refnum<user-event>, "Run VI":refnum<user-event>, "add_to_selection":refnum<user-event>, "clear_selection_list":refnum<user-event>, "remove_from_selection":refnum<user-event>, "enclose_selection":refnum<user-event>, "rename_object":refnum<user-event>, "set_value":refnum<user-event>, "delete_object":refnum<user-event>, "save_vi":refnum<user-event>, "get_structure_diagram":refnum<user-event>, "add_subvi":refnum<user-event>, "connect_to_pane":refnum<user-event>, "get_object_help":refnum<user-event>, "get_loop_conditional_terminal":refnum<user-event>, "show_conditional_terminal":refnum<user-event>, "get_loop_iteration_terminal":refnum<user-event>, "Read Config Data":refnum<user-event>, "get_allowed_paths":refnum<user-event>, "create_project":refnum<user-event>, "Set Allowed Paths":refnum<user-event>, "open_vi":refnum<user-event>}
  T2 = typedef "Scripting Server.lvlib/Module Data--cluster.ctl" = cluster{"Status":string, "Current ID":i32, "References":variant, "Config Data":T3}
  T3 = typedef "Scripting Server.lvlib/Config Data.ctl" = cluster{"Allowed Paths":string[]}
  T4 = enum32{"invalid lock state", "Not Locked", "Locked (No Password)", "Password-protected"}
  T5 = typedef "Scripting Server.lvlib/Stop Argument--cluster.ctl" = cluster{"Origin":string, "Exit via Stop Module Req?":bool, "Wait for Module to stop?":bool}
  T6 = typedef "Scripting Server.lvlib/New VI Argument--cluster.ctl" = cluster{"Open Frontpanel":bool, "Wait Notifier":refnum<notifier>, "wait for reply":bool}
  T7 = typedef "Scripting Server.lvlib/Add Object Argument--cluster.ctl" = cluster{"VI Reference":i32, "Object Name":string, "Wait Notifier":refnum<notifier>, "wait for reply":bool, "position_x":i32, "position_y":i32}
  T8 = typedef "Scripting Server.lvlib/Connect Objects Argument--cluster.ctl" = cluster{"vi reference":i32, "from object reference":i32, "to object reference":i32, "from object terminal index":i32, "to object terminal index":i32, "Wait Notifier":refnum<notifier>, "wait for reply":bool}
  T9 = typedef "Scripting Server.lvlib/Get Object Terminals Argument--cluster.ctl" = cluster{"object id":i32, "Wait Notifier":refnum<notifier>, "wait for reply":bool}
  T10 = typedef "Scripting Server.lvlib/get vi error list Argument--cluster.ctl" = cluster{"vi id":i32, "Wait Notifier":refnum<notifier>, "wait for reply":bool}
  T11 = typedef "Scripting Server.lvlib/Cleanup VI Argument--cluster.ctl" = cluster{"vi reference":i32, "Wait Notifier":refnum<notifier>, "wait for reply":bool}
  T12 = typedef "Scripting Server.lvlib/create_control Argument--cluster.ctl" = cluster{"Object ID":i32, "Terminal Index":i32, "Constant":bool, "Wait Notifier":refnum<notifier>, "wait for reply":bool, "Value":string}
  T13 = typedef "Scripting Server.lvlib/Run VI Argument--cluster.ctl" = cluster{"VI ID":i32, "open_frontpanel":bool, "Wait Notifier":refnum<notifier>, "wait for reply":bool}
  T14 = typedef "Scripting Server.lvlib/add_to_selection Argument--cluster.ctl" = cluster{"object_id":i32, "Wait Notifier":refnum<notifier>, "wait for reply":bool, "vi_id":i32}
  T15 = typedef "Scripting Server.lvlib/clear_selection_list Argument--cluster.ctl" = cluster{"Wait Notifier":refnum<notifier>, "wait for reply":bool, "vi_id":i32}
  T16 = typedef "Scripting Server.lvlib/remove_from_selection Argument--cluster.ctl" = cluster{"vi_id":i32, "object_id":i32, "Wait Notifier":refnum<notifier>, "wait for reply":bool}
  T17 = typedef "Scripting Server.lvlib/enclose_selection Argument--cluster.ctl" = cluster{"vi_id":i32, "structure_type":string, "Wait Notifier":refnum<notifier>, "wait for reply":bool}
  T18 = typedef "Scripting Server.lvlib/rename_object Argument--cluster.ctl" = cluster{"new_label_name":string, "label_visible":bool, "Wait Notifier":refnum<notifier>, "wait for reply":bool, "object_id":i32}
  T19 = typedef "Scripting Server.lvlib/set_value Argument--cluster.ctl" = cluster{"object_id":i32, "value":string, "Wait Notifier":refnum<notifier>, "wait for reply":bool}
  T20 = typedef "Scripting Server.lvlib/delete_object Argument--cluster.ctl" = cluster{"object_id":i32, "Wait Notifier":refnum<notifier>, "wait for reply":bool}
  T21 = typedef "Scripting Server.lvlib/save_vi Argument--cluster.ctl" = cluster{"vi_id":i32, "path":string, "Wait Notifier":refnum<notifier>, "wait for reply":bool}
  T22 = typedef "Scripting Server.lvlib/get_structure_diagram Argument--cluster.ctl" = cluster{"structure_id":i32, "index":i32, "Wait Notifier":refnum<notifier>, "wait for reply":bool}
  T23 = typedef "Scripting Server.lvlib/add_subvi Argument--cluster.ctl" = cluster{"diagram_id":i32, "subvi_path":string, "Wait Notifier":refnum<notifier>, "wait for reply":bool, "position_x":i32, "position_y":i32}
  T24 = typedef "Scripting Server.lvlib/connect_to_pane Argument--cluster.ctl" = cluster{"control_id":i32, "connector_pane_index":i32, "Wait Notifier":refnum<notifier>, "wait for reply":bool}
  T25 = typedef "Scripting Server.lvlib/get_object_help Argument--cluster.ctl" = cluster{"object_id":i32, "Wait Notifier":refnum<notifier>, "wait for reply":bool}
  T26 = typedef "Scripting Server.lvlib/get_loop_conditional_terminal Argument--cluster.ctl" = cluster{"loop_id":i32, "Wait Notifier":refnum<notifier>, "wait for reply":bool}
  T27 = typedef "Scripting Server.lvlib/show_conditional_terminal Argument--cluster.ctl" = cluster{"loop_id":i32, "show":bool, "Wait Notifier":refnum<notifier>, "wait for reply":bool}
  T28 = typedef "Scripting Server.lvlib/get_loop_iteration_terminal Argument--cluster.ctl" = cluster{"loop_id":i32, "Wait Notifier":refnum<notifier>, "wait for reply":bool}
  T29 = typedef "Scripting Server.lvlib/Read Config Data Argument--cluster.ctl" = cluster{"Boolean":bool}
  T30 = typedef "Scripting Server.lvlib/get_allowed_paths Argument--cluster.ctl" = cluster{"Wait Notifier":refnum<notifier>, "wait for reply":bool}
  T31 = typedef "Scripting Server.lvlib/create_project Argument--cluster.ctl" = cluster{"File Path":string, "Wait Notifier":refnum<notifier>, "wait for reply":bool}
  T32 = typedef "Scripting Server.lvlib/Set Allowed Paths Argument--cluster.ctl" = cluster{"Working Directory Folder Path":path[]}
  T33 = typedef "Scripting Server.lvlib/open_vi Argument--cluster.ctl" = cluster{"vi_path":string, "Wait Notifier":refnum<notifier>, "wait for reply":bool}
  T34 = typedef "LVPointTypeDef.ctl" = cluster{"Horizontal":i16, "Vertical":i16}
  T35 = enum32{"Invalid", "Standard", "Closed", "Hidden", "Minimized", "Maximized"}
  T36 = typedef "Scripting Server.lvlib/New VI (Reply Payload)--cluster.ctl" = cluster{"VI Reference":i32, "Result":string, "error":errorcluster}
  T37 = typedef "Scripting Server.lvlib/Add Object (Reply Payload)--cluster.ctl" = cluster{"error":errorcluster, "Object ID":i32, "Result":string}
  T38 = typedef "Scripting Server.lvlib/Connect Objects (Reply Payload)--cluster.ctl" = cluster{"result":string, "error":errorcluster}
  T39 = typedef "Scripting Server.lvlib/Get Object Terminals (Reply Payload)--cluster.ctl" = cluster{"terminals description":string, "error":errorcluster}
  T40 = typedef "Scripting Server.lvlib/get vi error list (Reply Payload)--cluster.ctl" = cluster{"error list":string, "error":errorcluster}
  T41 = typedef "Scripting Server.lvlib/create_control (Reply Payload)--cluster.ctl" = cluster{"Object ID":i32, "error":errorcluster}
  T42 = typedef "Scripting Server.lvlib/Run VI (Reply Payload)--cluster.ctl" = cluster{"error":errorcluster}
  T43 = typedef "Scripting Server.lvlib/add_to_selection (Reply Payload)--cluster.ctl" = cluster{"Current Selection":i32[], "error":errorcluster}
  T44 = typedef "Scripting Server.lvlib/clear_selection_list (Reply Payload)--cluster.ctl" = cluster{"error":errorcluster}
  T45 = typedef "Scripting Server.lvlib/remove_from_selection (Reply Payload)--cluster.ctl" = cluster{"current_selection":i32[], "error":errorcluster}
  T46 = typedef "Scripting Server.lvlib/enclose_selection (Reply Payload)--cluster.ctl" = cluster{"object_id":i32, "error":errorcluster}
  T47 = typedef "Scripting Server.lvlib/rename_object (Reply Payload)--cluster.ctl" = cluster{"error":errorcluster}
  T48 = typedef "Scripting Server.lvlib/set_value (Reply Payload)--cluster.ctl" = cluster{"error":errorcluster}
  T49 = typedef "Scripting Server.lvlib/delete_object (Reply Payload)--cluster.ctl" = cluster{"error":errorcluster}
  T50 = typedef "Scripting Server.lvlib/save_vi (Reply Payload)--cluster.ctl" = cluster{"path_out":string, "error":errorcluster}
  T51 = typedef "Scripting Server.lvlib/get_structure_diagram (Reply Payload)--cluster.ctl" = cluster{"diagram_id":i32, "error":errorcluster}
  T52 = typedef "Scripting Server.lvlib/add_subvi (Reply Payload)--cluster.ctl" = cluster{"subvi_id":i32, "error":errorcluster}
  T53 = typedef "Scripting Server.lvlib/connect_to_pane (Reply Payload)--cluster.ctl" = cluster{"error":errorcluster}
  T54 = typedef "Scripting Server.lvlib/get_object_help (Reply Payload)--cluster.ctl" = cluster{"help_string":string, "error":errorcluster}
  T55 = typedef "Scripting Server.lvlib/get_allowed_paths (Reply Payload)--cluster.ctl" = cluster{"Allowed Paths":string, "error":errorcluster}
  T56 = typedef "Scripting Server.lvlib/Cleanup VI (Reply Payload)--cluster.ctl" = cluster{"result":string, "error":errorcluster}
  T57 = typedef "Scripting Server.lvlib/get_loop_conditional_terminal (Reply Payload)--cluster.ctl" = cluster{"conditional_terminal_id":i32, "error":errorcluster}
  T58 = typedef "Scripting Server.lvlib/show_conditional_terminal (Reply Payload)--cluster.ctl" = cluster{"error":errorcluster}
  T59 = typedef "Scripting Server.lvlib/get_loop_iteration_terminal (Reply Payload)--cluster.ctl" = cluster{"iteration_terminal_id":i32, "error":errorcluster}
  T60 = typedef "Scripting Server.lvlib/create_project (Reply Payload)--cluster.ctl" = cluster{"project_id":i32, "error":errorcluster}
  T61 = typedef "Scripting Server.lvlib/open_vi (Reply Payload)--cluster.ctl" = cluster{"vi_id":string, "error":errorcluster}
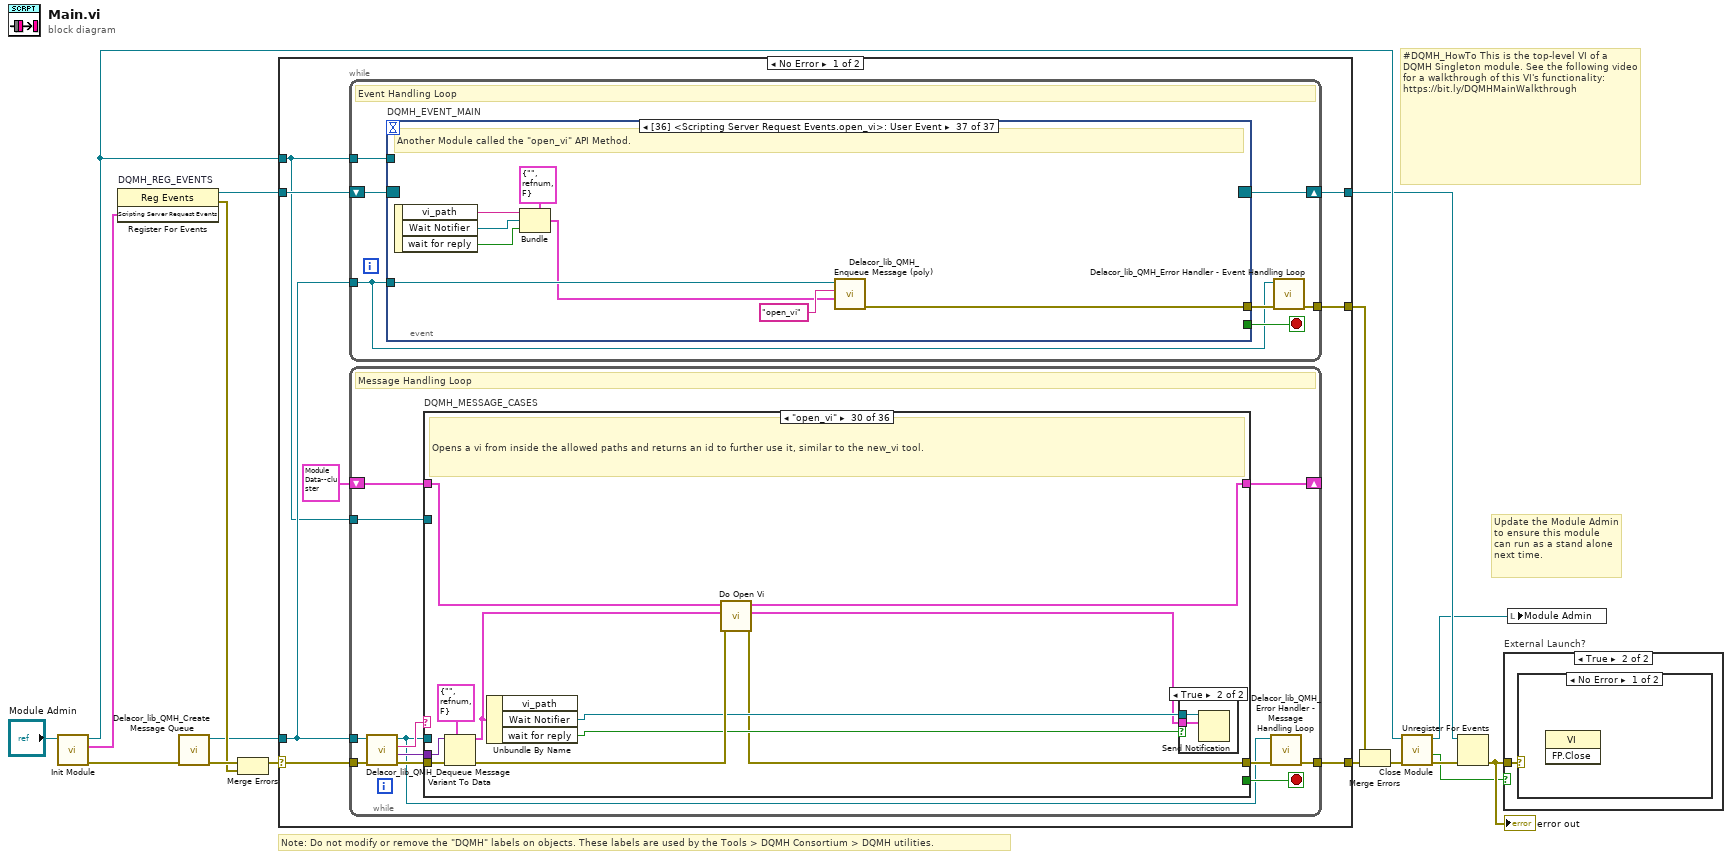
[diagram p0: block diagram]
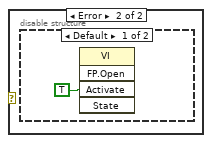
[diagram p3: hidden frame]
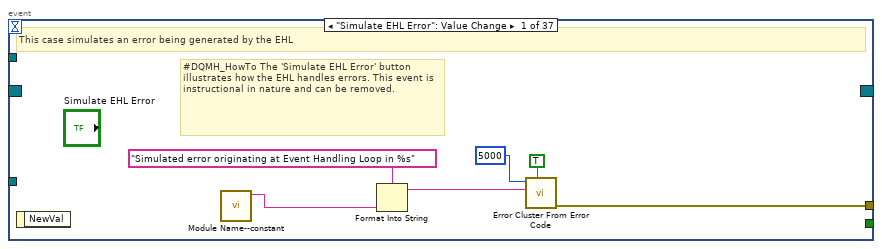
[diagram p5: hidden frame]
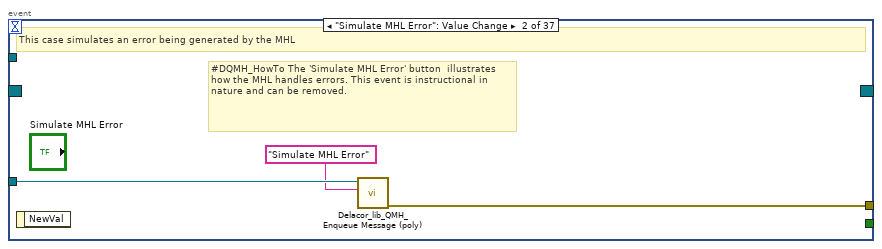
[diagram p6: hidden frame]
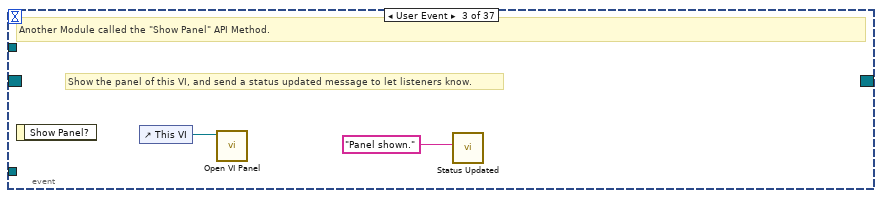
[diagram p7: hidden frame]
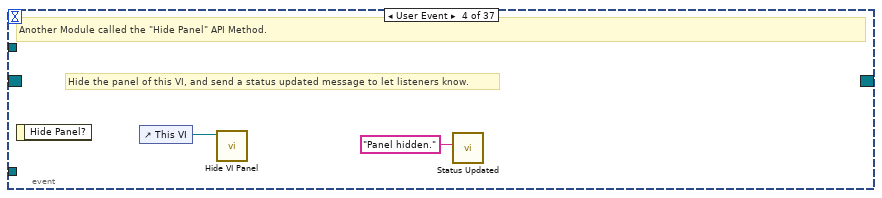
[diagram p8: hidden frame]
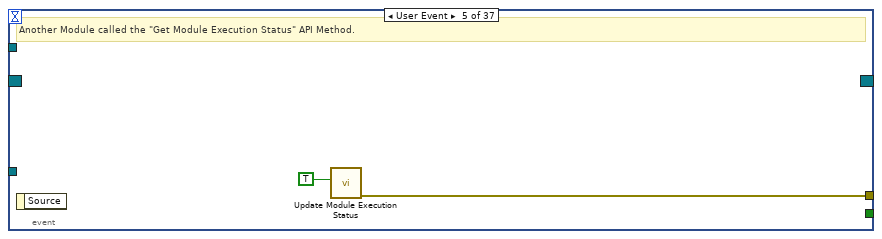
[diagram p9: hidden frame]
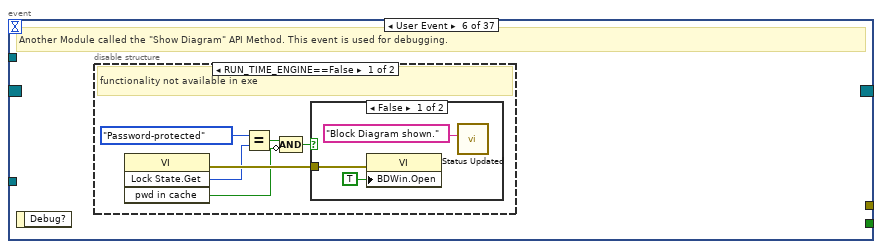
[diagram p10: hidden frame]
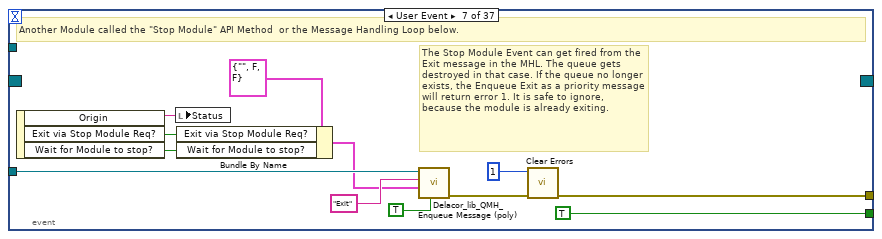
[diagram p13: hidden frame]
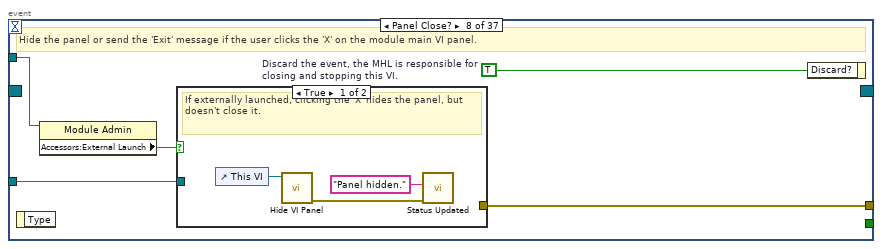
[diagram p14: hidden frame]
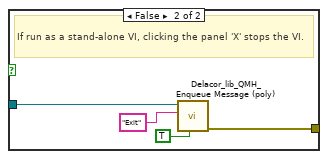
[diagram p15: hidden frame]
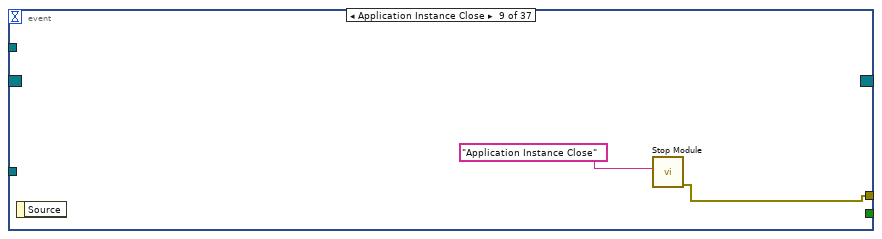
[diagram p16: hidden frame]
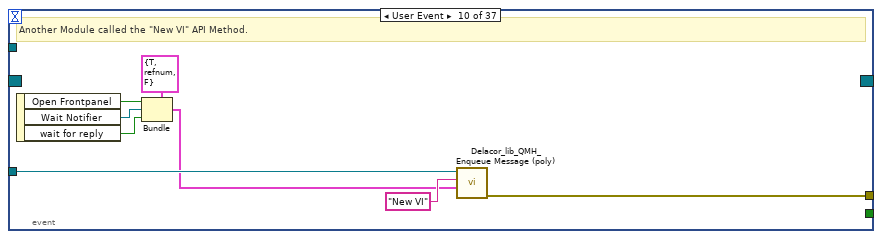
[diagram p17: hidden frame]
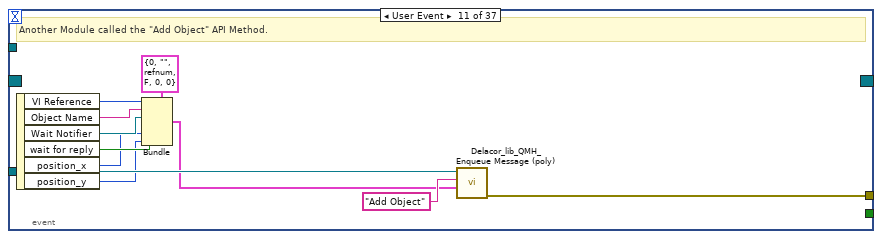
[diagram p18: hidden frame]
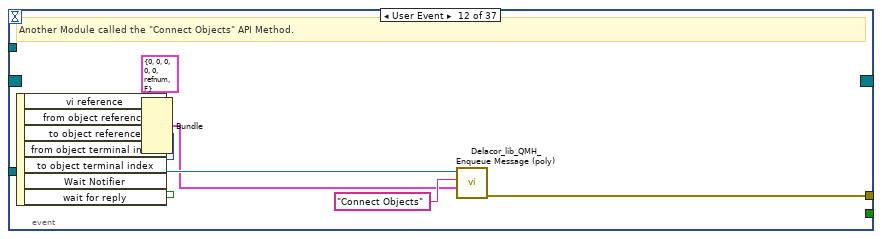
[diagram p19: hidden frame]
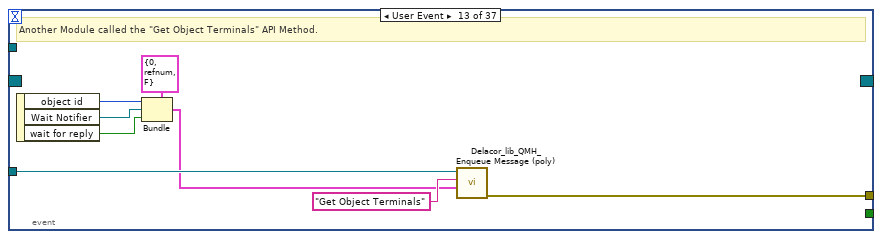
[diagram p20: hidden frame]
diagram:
  # "#DQMH_HowTo This is the top-level VI of a DQMH Singleton module. See the following video for a walkthrough of this VI's functionality: https://bit.ly/DQMHMainWalkthrough"
  # "Note: Do not modify or remove the \"DQMH\" labels on objects. These labels are used by the Tools > DQMH Consortium > DQMH utilities."
  # "Update the Module Admin to ensure this module can run as a stand alone next time."
  n1 = call "Init Module.vi"("Singleton Module Admin in"="Module Admin") -> ("error out"=w16:errorcluster, "Scripting Server Request Events"=w5:T1, "Singleton Module Admin out"=w8:refnum<class "Delacor_lib_QMH_Module Admin.lvclass">)  [unwired: 8 in]
  n2 = register-events "DQMH_REG_EVENTS"(w5) -> (reference out=w6:refnum<event-registration>, error out=w9:errorcluster)  [unwired: 2 in]
  n3 = call <vilib>:"Delacor_lib_QMH_Create Message Queue.vi"("error in"=w16) -> ("error out"=w11:errorcluster, "Message Queue"=w4:refnum<class "Delacor_lib_QMH_Message Queue.lvclass">)  [unwired: 9 in]
  n4 = Merge Errors(w11, w9) -> (w10:errorcluster)
  n5 = case shown="No Error" w10 {
    selector: w10 -> [w23 w817]
    tunnel: [w25 w816] -> w17
    tunnel: [w22 w815] -> w7
    tunnel: w6 -> [w20 w815]
    tunnel: w4 -> [w19 w810]
    tunnel: [w24 _] -> w14
    tunnel: w8 -> [w18 w811]
    frame No Error {
      n6 = while {
        tunnel: w19 -> [w26]
        shift-right: [w29] -> w22
        shift-left: w20 -> [w30]
        tunnel: [w31] -> w24
        tunnel: w18 -> [w27]
        stop <- w28 stop-if-true
        # "Event Handling Loop"
        n7 = event "DQMH_EVENT_MAIN" shown="[36] <Scripting Server Request Events.open_vi>: User Event" {
          selector: w30 -> [_ _ _ _ _ _ _ _ _ _ _ _ _ _ _ _ _ _ _ _ _ _ _ _ _ _ _ _ _ _ _ _ _ _ _ _ _]
          dyn-events: [_ _ _ _ _ _ _ _ _ _ _ _ _ _ _ _ _ _ _ _ _ _ _ _ _ _ _ _ _ _ _ _ _ _ _ _ _] -> w29
          timeout: _ -> [_ _ _ _ _ _ _ _ _ _ _ _ _ _ _ _ _ _ _ _ _ _ _ _ _ _ _ _ _ _ _ _ _ _ _ _ _]
          tunnel: [_ _ _ _ _ _ TRUE ("Discard?") _ _ _ _ _ _ _ _ _ _ _ _ _ _ _ _ _ _ _ _ _ _ _ _ _ _ _ _ _ _] -> w28
          tunnel: w26 -> [_ w40 _ _ _ _ w64 w71 _ w90 w101 w113 w121 w129 w137 w147 w156 w165 w173 w182 w191 w201 w210 w218 w227 w236 w245 w254 w262 w270 w279 w287 w293 w300 w308 w314 w322]
          tunnel: [w38 w41 _ _ w47 _ w67 w73 w82 w83 w95 w102 w114 w122 w130 w138 w148 w158 w167 w174 w183 w193 w202 w211 w219 w228 w237 w246 w255 w263 w271 w280 w288 w294 w301 w309 w315] -> w32
          tunnel: w27 -> [_ _ _ _ _ _ _ w70 _ _ _ _ _ _ _ _ _ _ _ _ _ _ _ _ _ _ _ _ _ _ _ _ _ _ _ _ _]
          event "Simulate EHL Error": Value Change {
            # "#DQMH_HowTo The 'Simulate EHL Error' button  illustrates how the EHL handles errors. This event is instructional in nature and can be removed."
            # "This case simulates an error being generated by the EHL"
            n8 = event-data() -> ()  [unwired: 1 in, 1 out]
            n9 = call "Module Name--constant.vi"() -> ("Module Name"=w35:string)  [unwired: 11 in]
            n10 = Format Into String(format string="Simulated error originating at Event Handling Loop in %s", w35) -> (resulting string=w36:string)  [unwired: 2 in, 1 out]
            n11 = call <vilib>:"Error Cluster From Error Code.vi"("show call chain? (False)"=TRUE, "error message (\"\")"=w36, "error code (0)"=5000) -> ("error out"=w38:errorcluster)  [unwired: 6 in]
          }
          event "Simulate MHL Error": Value Change {
            # "#DQMH_HowTo The 'Simulate MHL Error' button  illustrates how the MHL handles errors. This event is instructional in nature and can be removed."
            # "This case simulates an error being generated by the MHL"
            n12 = event-data() -> ()  [unwired: 1 in, 1 out]
            n13 = call-poly <vilib>:"Delacor_lib_QMH_Enqueue Message (poly).vi"("Message"="Simulate MHL Error", "Message Queue in"=w40) -> ("error out"=w41:errorcluster)  [unwired: 8 in, 1 out]
          }
          event User Event {
            # "Show the panel of this VI, and send a status updated message to let listeners know."
            # "Another Module called the \"Show Panel\" API Method."
            n14 = event-data() -> ()  [unwired: 1 in, 1 out]
            n15 = control-ref of="This VI"() -> (w43:refnum<vi>)
            n16 = call "Open VI Panel.vi"("VI"=w43) -> ()  [unwired: 10 in, 1 out]
            n17 = call "Status Updated.vi"("Status"="Panel shown." ("format string")) -> ()  [unwired: 10 in, 1 out]
          }
          event User Event {
            # "Hide the panel of this VI, and send a status updated message to let listeners know."
            # "Another Module called the \"Hide Panel\" API Method."
            n18 = event-data() -> ()  [unwired: 1 in, 1 out]
            n19 = control-ref of="This VI"() -> (w45:refnum<vi>)
            n20 = call "Hide VI Panel.vi"("VI"=w45) -> ()  [unwired: 10 in, 1 out]
            n21 = call "Status Updated.vi"("Status"="Panel hidden." ("format string")) -> ()  [unwired: 10 in, 1 out]
          }
          event User Event {
            # "Another Module called the \"Get Module Execution Status\" API Method."
            n22 = event-data() -> ()  [unwired: 1 in, 1 out]
            n23 = call "Update Module Execution Status.vi"("Running?"=TRUE) -> ("error out"=w47:errorcluster)  [unwired: 10 in]
          }
          event User Event {
            # "Another Module called the \"Show Diagram\" API Method. This event is used for debugging."
            n24 = event-data() -> ()  [unwired: 1 in, 1 out]
            n25 = disable-structure shown="RUN_TIME_ENGINE==False" {
              frame condition #0 (active) {
                # "functionality not available in exe"
                n26 = invoke on="Invoke Node" class="VI" method="Lock State.Get"() -> (error out=w53:errorcluster, "Get Lock State"=w52:T4, "pwd in cache"=w49:bool)  [unwired: 4 in, 1 out]
                n27 = Equal?(x=T4."Password-protected", y=w52) -> (x = y?=w50:bool)
                n28 = Compound Arithmetic op=AND(w50, invert w49) -> (w48:bool)
                n29 = case shown="False" w48 {
                  tunnel: w53 -> [w56 _]
                  frame False {
                    n30 = property on="Property Node" class="VI"(error in=w56, "BDWin.Open"=TRUE ("Block Diagram Window:Open")) -> ()  [unwired: 1 in, 2 out]
                    n31 = call "Status Updated.vi"("Status"="Block Diagram shown." ("format string")) -> ()  [unwired: 10 in, 1 out]
                  }
                  frame True {
                    # "Password-protected VI, and the password is not in the cache. Do not show the diagram."
                  }
                }
              }
              frame condition #1 {
              }
            }
          }
          event User Event {
            # "The Stop Module Event can get fired from the Exit message in the MHL. The queue gets destroyed in that case. If the queue no longer exists, the Enqueue Exit as a priority message will return error 1. It is safe to ignore, because the module is already exiting."
            # "Another Module called the \"Stop Module\" API Method  or the Message Handling Loop below."
            n32 = event-data() -> ("Origin"=w63:string, "Exit via Stop Module Req?"=w59:bool, "Wait for Module to stop?"=w58:bool)  [unwired: 1 in]
            n33 = local write "Status"(w63) -> ()
            n34 = Bundle By Name(cluster=T5 {"Origin"="", "Exit via Stop Module Req?"=FALSE, "Wait for Module to stop?"=FALSE} ("Stop Argument"), "Exit via Stop Module Req?"=w59, "Wait for Module to stop?"=w58) -> (w57:T5)
            n35 = call-poly <vilib>:"Delacor_lib_QMH_Enqueue Message (poly).vi"("Priority Message? (F)"=TRUE, "Message Data"=w57, "Message"="Exit", "Message Queue in"=w64) -> ("error out"=w68:errorcluster)  [unwired: 6 in, 1 out]
            n36 = call <vilib>:"Clear Errors.vi"("error in (no error)"=w68, "specific error code to clear (0: all)"=1) -> ("error out"=w67:errorcluster)  [unwired: 4 in, 1 out]
          }
          event Panel Close? {
            w72 = TRUE  # Discard the event, the MHL is responsible for closing and stopping this VI.
            # "Hide the panel or send the 'Exit' message if the user clicks the 'X' on the module main VI panel."
            n37 = event-data() -> ()  [unwired: 1 in, 1 out]
            n38 = property on="Property Node" class="Module Admin"(reference=w70) -> ("Accessors:External Launch"=w69:bool)  [unwired: 1 in, 2 out]
            n39 = case shown="True" w69 {
              tunnel: w71 -> [_ w79]
              tunnel: [_ w80] -> w73
              frame True {
                # "If externally launched, clicking the 'X' hides the panel, but doesn't close it."
                n40 = control-ref of="This VI"() -> (w76:refnum<vi>)
                n41 = call "Hide VI Panel.vi"("VI"=w76) -> ("error out"=w74:errorcluster)  [unwired: 10 in]
                n42 = call "Status Updated.vi"("error in"=w74, "Status"="Panel hidden." ("format string")) -> ()  [unwired: 9 in, 1 out]
              }
              frame False {
                # "If run as a stand-alone VI, clicking the panel 'X' stops the VI."
                n43 = call-poly <vilib>:"Delacor_lib_QMH_Enqueue Message (poly).vi"("Priority Message? (F)"=TRUE, "Message"="Exit", "Message Queue in"=w79) -> ("error out"=w80:errorcluster)  [unwired: 7 in, 1 out]
              }
            }
            n44 = event-data ("Event Filter Node")("Discard?"=w72) -> ()  [unwired: 1 in, 1 out]
          }
          event Application Instance Close {
            n45 = event-data() -> ()  [unwired: 1 in, 1 out]
            n46 = call "Stop Module.vi"("Origin"="Application Instance Close") -> ("error out"=w82:errorcluster)  [unwired: 10 in]
          }
          event User Event {
            # "Another Module called the \"New VI\" API Method."
            n47 = event-data() -> ("Open Frontpanel"=w86:bool, "Wait Notifier"=w85:refnum<notifier>, "wait for reply"=w84:bool)  [unwired: 1 in]
            n48 = Bundle(cluster=T6 {"Open Frontpanel"=TRUE, "Wait Notifier"=refnum, "wait for reply"=FALSE} ("New VI Argument"), "Open Frontpanel"=w86, "Wait Notifier"=w85, "wait for reply"=w84) -> (w87:T6)
            n49 = call-poly <vilib>:"Delacor_lib_QMH_Enqueue Message (poly).vi"("Message Data"=w87, "Message"="New VI", "Message Queue in"=w90) -> ("error out"=w83:errorcluster)  [unwired: 7 in, 1 out]
          }
          event User Event {
            # "Another Module called the \"Add Object\" API Method."
            n50 = event-data() -> ("VI Reference"=w97:i32, "Object Name"=w96:string, "Wait Notifier"=w94:refnum<notifier>, "wait for reply"=w93:bool, "position_x"=w92:i32, "position_y"=w91:i32)  [unwired: 1 in]
            n51 = Bundle(cluster=T7 {"VI Reference"=0, "Object Name"="", "Wait Notifier"=refnum, "wait for reply"=FALSE, "position_x"=0, "position_y"=0} ("Add Object Argument"), "VI Reference"=w97, "Object Name"=w96, "Wait Notifier"=w94, "wait for reply"=w93, "position_x"=w92, "position_y"=w91) -> (w98:T7)
            n52 = call-poly <vilib>:"Delacor_lib_QMH_Enqueue Message (poly).vi"("Message Data"=w98, "Message"="Add Object", "Message Queue in"=w101) -> ("error out"=w95:errorcluster)  [unwired: 7 in, 1 out]
          }
          event User Event {
            # "Another Module called the \"Connect Objects\" API Method."
            n53 = event-data() -> ("vi reference"=w109:i32, "from object reference"=w108:i32, "to object reference"=w107:i32, "from object terminal index"=w106:i32, "to object terminal index"=w105:i32, "Wait Notifier"=w104:refnum<notifier>, "wait for reply"=w103:bool)  [unwired: 1 in]
            n54 = Bundle(cluster=T8 {"vi reference"=0, "from object reference"=0, "to object reference"=0, "from object terminal index"=0, "to object terminal index"=0, "Wait Notifier"=refnum, "wait for reply"=FALSE} ("Connect Objects Argument"), "vi reference"=w109, "from object reference"=w108, "to object reference"=w107, "from object terminal index"=w106, "to object terminal index"=w105, "Wait Notifier"=w104, "wait for reply"=w103) -> (w110:T8)
            n55 = call-poly <vilib>:"Delacor_lib_QMH_Enqueue Message (poly).vi"("Message Data"=w110, "Message"="Connect Objects", "Message Queue in"=w113) -> ("error out"=w102:errorcluster)  [unwired: 7 in, 1 out]
          }
          event User Event {
            # "Another Module called the \"Get Object Terminals\" API Method."
            n56 = event-data() -> ("object id"=w117:i32, "Wait Notifier"=w116:refnum<notifier>, "wait for reply"=w115:bool)  [unwired: 1 in]
            n57 = Bundle(cluster=T9 {"object id"=0, "Wait Notifier"=refnum, "wait for reply"=FALSE} ("Get Object Terminals Argument"), "object id"=w117, "Wait Notifier"=w116, "wait for reply"=w115) -> (w118:T9)
            n58 = call-poly <vilib>:"Delacor_lib_QMH_Enqueue Message (poly).vi"("Message Data"=w118, "Message"="Get Object Terminals", "Message Queue in"=w121) -> ("error out"=w114:errorcluster)  [unwired: 7 in, 1 out]
          }
          event User Event {
            # "Another Module called the \"get vi error list\" API Method."
            n59 = event-data() -> ("vi id"=w125:i32, "Wait Notifier"=w124:refnum<notifier>, "wait for reply"=w123:bool)  [unwired: 1 in]
            n60 = Bundle(cluster=T10 {"vi id"=0, "Wait Notifier"=refnum, "wait for reply"=FALSE} ("get vi error list Argument"), "vi id"=w125, "Wait Notifier"=w124, "wait for reply"=w123) -> (w126:T10)
            n61 = call-poly <vilib>:"Delacor_lib_QMH_Enqueue Message (poly).vi"("Message Data"=w126, "Message"="get vi error list", "Message Queue in"=w129) -> ("error out"=w122:errorcluster)  [unwired: 7 in, 1 out]
          }
          event User Event {
            # "Another Module called the \"Cleanup VI\" API Method."
            n62 = event-data() -> ("vi reference"=w133:i32, "Wait Notifier"=w132:refnum<notifier>, "wait for reply"=w131:bool)  [unwired: 1 in]
            n63 = Bundle(cluster=T11 {"vi reference"=0, "Wait Notifier"=refnum, "wait for reply"=FALSE} ("Cleanup VI Argument"), "vi reference"=w133, "Wait Notifier"=w132, "wait for reply"=w131) -> (w134:T11)
            n64 = call-poly <vilib>:"Delacor_lib_QMH_Enqueue Message (poly).vi"("Message Data"=w134, "Message"="Cleanup VI", "Message Queue in"=w137) -> ("error out"=w130:errorcluster)  [unwired: 7 in, 1 out]
          }
          event User Event {
            # "Another Module called the \"create_control\" API Method."
            n65 = event-data() -> ("Object ID"=w143:i32, "Terminal Index"=w142:i32, "Constant"=w141:bool, "Wait Notifier"=w140:refnum<notifier>, "wait for reply"=w139:bool)  [unwired: 1 in]
            n66 = Bundle(cluster=T12 {"Object ID"=0, "Terminal Index"=0, "Constant"=FALSE, "Wait Notifier"=refnum, "wait for reply"=FALSE, "Value"=""} ("create_control Argument"), "Object ID"=w143, "Terminal Index"=w142, "Constant"=w141, "Wait Notifier"=w140, "wait for reply"=w139) -> (w144:T12)  [unwired: 1 in]
            n67 = call-poly <vilib>:"Delacor_lib_QMH_Enqueue Message (poly).vi"("Message Data"=w144, "Message"="create_control", "Message Queue in"=w147) -> ("error out"=w138:errorcluster)  [unwired: 7 in, 1 out]
          }
          event User Event {
            # "Another Module called the \"Run VI\" API Method."
            n68 = event-data() -> ("VI ID"=w152:i32, "open_frontpanel"=w151:bool, "Wait Notifier"=w150:refnum<notifier>, "wait for reply"=w149:bool)  [unwired: 1 in]
            n69 = Bundle(cluster=T13 {"VI ID"=0, "open_frontpanel"=FALSE, "Wait Notifier"=refnum, "wait for reply"=FALSE} ("Run VI Argument"), "VI ID"=w152, "open_frontpanel"=w151, "Wait Notifier"=w150, "wait for reply"=w149) -> (w153:T13)
            n70 = call-poly <vilib>:"Delacor_lib_QMH_Enqueue Message (poly).vi"("Message Data"=w153, "Message"="Run VI", "Message Queue in"=w156) -> ("error out"=w148:errorcluster)  [unwired: 7 in, 1 out]
          }
          event User Event {
            # "Another Module called the \"add_to_selection\" API Method."
            n71 = event-data() -> ("object_id"=w161:i32, "Wait Notifier"=w160:refnum<notifier>, "wait for reply"=w159:bool, "vi_id"=w157:i32)  [unwired: 1 in]
            n72 = Bundle(cluster=T14 {"object_id"=0, "Wait Notifier"=refnum, "wait for reply"=FALSE, "vi_id"=0} ("add_to_selection Argument"), "object_id"=w161, "Wait Notifier"=w160, "wait for reply"=w159, "vi_id"=w157) -> (w162:T14)
            n73 = call-poly <vilib>:"Delacor_lib_QMH_Enqueue Message (poly).vi"("Message Data"=w162, "Message"="add_to_selection", "Message Queue in"=w165) -> ("error out"=w158:errorcluster)  [unwired: 7 in, 1 out]
          }
          event User Event {
            # "Another Module called the \"clear_selection_list\" API Method."
            n74 = event-data() -> ("Wait Notifier"=w169:refnum<notifier>, "wait for reply"=w168:bool, "vi_id"=w166:i32)  [unwired: 1 in]
            n75 = Bundle(cluster=T15 {"Wait Notifier"=refnum, "wait for reply"=FALSE, "vi_id"=0} ("clear_selection_list Argument"), "Wait Notifier"=w169, "wait for reply"=w168, "vi_id"=w166) -> (w170:T15)
            n76 = call-poly <vilib>:"Delacor_lib_QMH_Enqueue Message (poly).vi"("Message Data"=w170, "Message"="clear_selection_list", "Message Queue in"=w173) -> ("error out"=w167:errorcluster)  [unwired: 7 in, 1 out]
          }
          event User Event {
            # "Another Module called the \"remove_from_selection\" API Method."
            n77 = event-data() -> ("vi_id"=w178:i32, "object_id"=w177:i32, "Wait Notifier"=w176:refnum<notifier>, "wait for reply"=w175:bool)  [unwired: 1 in]
            n78 = Bundle(cluster=T16 {"vi_id"=0, "object_id"=0, "Wait Notifier"=refnum, "wait for reply"=FALSE} ("remove_from_selection Argument"), "vi_id"=w178, "object_id"=w177, "Wait Notifier"=w176, "wait for reply"=w175) -> (w179:T16)
            n79 = call-poly <vilib>:"Delacor_lib_QMH_Enqueue Message (poly).vi"("Message Data"=w179, "Message"="remove_from_selection", "Message Queue in"=w182) -> ("error out"=w174:errorcluster)  [unwired: 7 in, 1 out]
          }
          event User Event {
            # "Another Module called the \"enclose_selection\" API Method."
            n80 = event-data() -> ("vi_id"=w187:i32, "structure_type"=w186:string, "Wait Notifier"=w185:refnum<notifier>, "wait for reply"=w184:bool)  [unwired: 1 in]
            n81 = Bundle(cluster=T17 {"vi_id"=0, "structure_type"="", "Wait Notifier"=refnum, "wait for reply"=FALSE} ("enclose_selection Argument"), "vi_id"=w187, "structure_type"=w186, "Wait Notifier"=w185, "wait for reply"=w184) -> (w188:T17)
            n82 = call-poly <vilib>:"Delacor_lib_QMH_Enqueue Message (poly).vi"("Message Data"=w188, "Message"="enclose_selection", "Message Queue in"=w191) -> ("error out"=w183:errorcluster)  [unwired: 7 in, 1 out]
          }
          event User Event {
            # "Another Module called the \"rename_object\" API Method."
            n83 = event-data() -> ("new_label_name"=w197:string, "label_visible"=w196:bool, "Wait Notifier"=w195:refnum<notifier>, "wait for reply"=w194:bool, "object_id"=w192:i32)  [unwired: 1 in]
            n84 = Bundle(cluster=T18 {"new_label_name"="", "label_visible"=FALSE, "Wait Notifier"=refnum, "wait for reply"=FALSE, "object_id"=0} ("rename_object Argument"), "new_label_name"=w197, "label_visible"=w196, "Wait Notifier"=w195, "wait for reply"=w194, "object_id"=w192) -> (w198:T18)
            n85 = call-poly <vilib>:"Delacor_lib_QMH_Enqueue Message (poly).vi"("Message Data"=w198, "Message"="rename_object", "Message Queue in"=w201) -> ("error out"=w193:errorcluster)  [unwired: 7 in, 1 out]
          }
          event User Event {
            # "Another Module called the \"set_value\" API Method."
            n86 = event-data() -> ("object_id"=w206:i32, "value"=w205:string, "Wait Notifier"=w204:refnum<notifier>, "wait for reply"=w203:bool)  [unwired: 1 in]
            n87 = Bundle(cluster=T19 {"object_id"=0, "value"="", "Wait Notifier"=refnum, "wait for reply"=FALSE} ("set_value Argument"), "object_id"=w206, "value"=w205, "Wait Notifier"=w204, "wait for reply"=w203) -> (w207:T19)
            n88 = call-poly <vilib>:"Delacor_lib_QMH_Enqueue Message (poly).vi"("Message Data"=w207, "Message"="set_value", "Message Queue in"=w210) -> ("error out"=w202:errorcluster)  [unwired: 7 in, 1 out]
          }
          event User Event {
            # "Another Module called the \"delete_object\" API Method."
            n89 = event-data() -> ("object_id"=w214:i32, "Wait Notifier"=w213:refnum<notifier>, "wait for reply"=w212:bool)  [unwired: 1 in]
            n90 = Bundle(cluster=T20 {"object_id"=0, "Wait Notifier"=refnum, "wait for reply"=FALSE} ("delete_object Argument"), "object_id"=w214, "Wait Notifier"=w213, "wait for reply"=w212) -> (w215:T20)
            n91 = call-poly <vilib>:"Delacor_lib_QMH_Enqueue Message (poly).vi"("Message Data"=w215, "Message"="delete_object", "Message Queue in"=w218) -> ("error out"=w211:errorcluster)  [unwired: 7 in, 1 out]
          }
          event User Event {
            # "Another Module called the \"save_vi\" API Method."
            n92 = event-data() -> ("vi_id"=w223:i32, "path"=w222:string, "Wait Notifier"=w221:refnum<notifier>, "wait for reply"=w220:bool)  [unwired: 1 in]
            n93 = Bundle(cluster=T21 {"vi_id"=0, "path"="", "Wait Notifier"=refnum, "wait for reply"=FALSE} ("save_vi Argument"), "vi_id"=w223, "path"=w222, "Wait Notifier"=w221, "wait for reply"=w220) -> (w224:T21)
            n94 = call-poly <vilib>:"Delacor_lib_QMH_Enqueue Message (poly).vi"("Message Data"=w224, "Message"="save_vi", "Message Queue in"=w227) -> ("error out"=w219:errorcluster)  [unwired: 7 in, 1 out]
          }
          event User Event {
            # "Another Module called the \"get_structure_diagram\" API Method."
            n95 = event-data() -> ("structure_id"=w232:i32, "index"=w231:i32, "Wait Notifier"=w230:refnum<notifier>, "wait for reply"=w229:bool)  [unwired: 1 in]
            n96 = Bundle(cluster=T22 {"structure_id"=0, "index"=0, "Wait Notifier"=refnum, "wait for reply"=FALSE} ("get_structure_diagram Argument"), "structure_id"=w232, "index"=w231, "Wait Notifier"=w230, "wait for reply"=w229) -> (w233:T22)
            n97 = call-poly <vilib>:"Delacor_lib_QMH_Enqueue Message (poly).vi"("Message Data"=w233, "Message"="get_structure_diagram", "Message Queue in"=w236) -> ("error out"=w228:errorcluster)  [unwired: 7 in, 1 out]
          }
          event User Event {
            # "Another Module called the \"add_subvi\" API Method."
            n98 = event-data() -> ("diagram_id"=w241:i32, "subvi_path"=w240:string, "Wait Notifier"=w239:refnum<notifier>, "wait for reply"=w238:bool)  [unwired: 1 in]
            n99 = Bundle(cluster=T23 {"diagram_id"=0, "subvi_path"="", "Wait Notifier"=refnum, "wait for reply"=FALSE, "position_x"=0, "position_y"=0} ("add_subvi Argument"), "diagram_id"=w241, "subvi_path"=w240, "Wait Notifier"=w239, "wait for reply"=w238) -> (w242:T23)  [unwired: 2 in]
            n100 = call-poly <vilib>:"Delacor_lib_QMH_Enqueue Message (poly).vi"("Message Data"=w242, "Message"="add_subvi", "Message Queue in"=w245) -> ("error out"=w237:errorcluster)  [unwired: 7 in, 1 out]
          }
          event User Event {
            # "Another Module called the \"connect_to_pane\" API Method."
            n101 = event-data() -> ("control_id"=w250:i32, "connector_pane_index"=w249:i32, "Wait Notifier"=w248:refnum<notifier>, "wait for reply"=w247:bool)  [unwired: 1 in]
            n102 = Bundle(cluster=T24 {"control_id"=0, "connector_pane_index"=0, "Wait Notifier"=refnum, "wait for reply"=FALSE} ("connect_to_pane Argument"), "control_id"=w250, "connector_pane_index"=w249, "Wait Notifier"=w248, "wait for reply"=w247) -> (w251:T24)
            n103 = call-poly <vilib>:"Delacor_lib_QMH_Enqueue Message (poly).vi"("Message Data"=w251, "Message"="connect_to_pane", "Message Queue in"=w254) -> ("error out"=w246:errorcluster)  [unwired: 7 in, 1 out]
          }
          event User Event {
            # "Another Module called the \"get_object_help\" API Method."
            n104 = event-data() -> ("object_id"=w258:i32, "Wait Notifier"=w257:refnum<notifier>, "wait for reply"=w256:bool)  [unwired: 1 in]
            n105 = Bundle(cluster=T25 {"object_id"=0, "Wait Notifier"=refnum, "wait for reply"=FALSE} ("get_object_help Argument"), "object_id"=w258, "Wait Notifier"=w257, "wait for reply"=w256) -> (w259:T25)
            n106 = call-poly <vilib>:"Delacor_lib_QMH_Enqueue Message (poly).vi"("Message Data"=w259, "Message"="get_object_help", "Message Queue in"=w262) -> ("error out"=w255:errorcluster)  [unwired: 7 in, 1 out]
          }
          event User Event {
            # "Another Module called the \"get_loop_conditional_terminal\" API Method."
            n107 = event-data() -> ("loop_id"=w266:i32, "Wait Notifier"=w265:refnum<notifier>, "wait for reply"=w264:bool)  [unwired: 1 in]
            n108 = Bundle(cluster=T26 {"loop_id"=0, "Wait Notifier"=refnum, "wait for reply"=FALSE} ("get_loop_conditional_terminal Argument"), "loop_id"=w266, "Wait Notifier"=w265, "wait for reply"=w264) -> (w267:T26)
            n109 = call-poly <vilib>:"Delacor_lib_QMH_Enqueue Message (poly).vi"("Message Data"=w267, "Message"="get_loop_conditional_terminal", "Message Queue in"=w270) -> ("error out"=w263:errorcluster)  [unwired: 7 in, 1 out]
          }
          event User Event {
            # "Another Module called the \"show_conditional_terminal\" API Method."
            n110 = event-data() -> ("loop_id"=w275:i32, "show"=w274:bool, "Wait Notifier"=w273:refnum<notifier>, "wait for reply"=w272:bool)  [unwired: 1 in]
            n111 = Bundle(cluster=T27 {"loop_id"=0, "show"=FALSE, "Wait Notifier"=refnum, "wait for reply"=FALSE} ("show_conditional_terminal Argument"), "loop_id"=w275, "show"=w274, "Wait Notifier"=w273, "wait for reply"=w272) -> (w276:T27)
            n112 = call-poly <vilib>:"Delacor_lib_QMH_Enqueue Message (poly).vi"("Message Data"=w276, "Message"="show_conditional_terminal", "Message Queue in"=w279) -> ("error out"=w271:errorcluster)  [unwired: 7 in, 1 out]
          }
          event User Event {
            # "Another Module called the \"get_loop_iteration_terminal\" API Method."
            n113 = event-data() -> ("loop_id"=w283:i32, "Wait Notifier"=w282:refnum<notifier>, "wait for reply"=w281:bool)  [unwired: 1 in]
            n114 = Bundle(cluster=T28 {"loop_id"=0, "Wait Notifier"=refnum, "wait for reply"=FALSE} ("get_loop_iteration_terminal Argument"), "loop_id"=w283, "Wait Notifier"=w282, "wait for reply"=w281) -> (w284:T28)
            n115 = call-poly <vilib>:"Delacor_lib_QMH_Enqueue Message (poly).vi"("Message Data"=w284, "Message"="get_loop_iteration_terminal", "Message Queue in"=w287) -> ("error out"=w280:errorcluster)  [unwired: 7 in, 1 out]
          }
          event User Event {
            # "Another Module called the \"Read Config Data\" API Method."
            n116 = event-data() -> ("Boolean"=w289:bool)  [unwired: 1 in]
            n117 = Bundle(cluster=T29 {"Boolean"=FALSE} ("Read Config Data Argument"), "Boolean"=w289) -> (w290:T29)
            n118 = call-poly <vilib>:"Delacor_lib_QMH_Enqueue Message (poly).vi"("Message Data"=w290, "Message"="Read Config Data", "Message Queue in"=w293) -> ("error out"=w288:errorcluster)  [unwired: 7 in, 1 out]
          }
          event User Event {
            # "Another Module called the \"get_allowed_paths\" API Method."
            n119 = event-data() -> ("Wait Notifier"=w296:refnum<notifier>, "wait for reply"=w295:bool)  [unwired: 1 in]
            n120 = Bundle(cluster=T30 {"Wait Notifier"=refnum, "wait for reply"=FALSE} ("get_allowed_paths Argument"), "Wait Notifier"=w296, "wait for reply"=w295) -> (w297:T30)
            n121 = call-poly <vilib>:"Delacor_lib_QMH_Enqueue Message (poly).vi"("Message Data"=w297, "Message"="get_allowed_paths", "Message Queue in"=w300) -> ("error out"=w294:errorcluster)  [unwired: 7 in, 1 out]
          }
          event User Event {
            # "Another Module called the \"create_project\" API Method."
            n122 = event-data() -> ("File Path"=w304:string, "Wait Notifier"=w303:refnum<notifier>, "wait for reply"=w302:bool)  [unwired: 1 in]
            n123 = Bundle(cluster=T31 {"File Path"="", "Wait Notifier"=refnum, "wait for reply"=FALSE} ("create_project Argument"), "File Path"=w304, "Wait Notifier"=w303, "wait for reply"=w302) -> (w305:T31)
            n124 = call-poly <vilib>:"Delacor_lib_QMH_Enqueue Message (poly).vi"("Message Data"=w305, "Message"="create_project", "Message Queue in"=w308) -> ("error out"=w301:errorcluster)  [unwired: 7 in, 1 out]
          }
          event User Event {
            # "Another Module called the \"Set Allowed Paths\" API Method."
            n125 = event-data() -> ("Working Directory Folder Path"=w310:path[])  [unwired: 1 in]
            n126 = Bundle(cluster=T32 {"Working Directory Folder Path"=[]} ("Set Working Directory Argument"), "Working Directory Folder Path"=w310) -> (w311:T32)
            n127 = call-poly <vilib>:"Delacor_lib_QMH_Enqueue Message (poly).vi"("Message Data"=w311, "Message"="Set Working Directory", "Message Queue in"=w314) -> ("error out"=w309:errorcluster)  [unwired: 7 in, 1 out]
          }
          event User Event {
            # "Another Module called the \"open_vi\" API Method."
            n128 = event-data() -> ("vi_path"=w318:string, "Wait Notifier"=w317:refnum<notifier>, "wait for reply"=w316:bool)  [unwired: 1 in]
            n129 = Bundle(cluster=T33 {"vi_path"="", "Wait Notifier"=refnum, "wait for reply"=FALSE} ("open_vi Argument"), "vi_path"=w318, "Wait Notifier"=w317, "wait for reply"=w316) -> (w319:T33)
            n130 = call-poly <vilib>:"Delacor_lib_QMH_Enqueue Message (poly).vi"("Message Data"=w319, "Message"="open_vi", "Message Queue in"=w322) -> ("error out"=w315:errorcluster)  [unwired: 7 in, 1 out]
          }
        }
        n131 = call-dynamic "Delacor_lib_QMH_Error Handler - Event Handling Loop.vi"("error in"=w32, "Message Queue in"=w26) -> ("dup error in"=w31:errorcluster)  [unwired: 8 in, 1 out]
      }
      n132 = while {
        tunnel: w19 -> [w323]
        shift-right: [w331] -> _
        shift-left: T2 {"Status"="", "Current ID"=0, "References"=variant, "Config Data"={"Allowed Paths"=[]}} ("Data Cluster") -> [w332]
        tunnel: w23 -> [w334]
        tunnel: [w326] -> w25
        tunnel: w18 -> [w327]
        stop <- w330 stop-if-true
        # "Message Handling Loop"
        n133 = call-dynamic "Delacor_lib_QMH_Dequeue Message.vi"("error in"=w334, "Message Queue in"=w323) -> ("error out"=w333:errorcluster, "Message Data"=w328:variant, "Message"=w329:string, "Message Queue out"=w324:refnum<class "Delacor_lib_QMH_Message Queue.lvclass">)  [unwired: 6 in]
        n134 = case "DQMH_MESSAGE_CASES" shown="\"open_vi\"" w329 {
          selector: w329 -> [_ _ _ _ _ _ _ _ _ _ _ _ _ _ _ _ _ _ _ _ _ _ _ _ _ _ _ _ _ _ _ _ _ _ _ w805]
          tunnel: w324 -> [_ _ _ _ _ _ _ _ _ _ _ _ _ _ _ _ _ _ _ _ _ _ _ _ _ _ _ _ _ _ _ _ _ w771 w793 _]
          tunnel: w333 -> [w353 w357 w372 w389 w403 w418 w433 w445 w460 w474 w488 w502 w516 w531 w545 w559 w573 w589 w604 w619 w633 w648 w661 w674 w687 w701 w713 w729 w740 w751 w756 w758 w767 w778 w799 w808]
          tunnel: [w351 w357 w363 w377 w392 w406 w421 w436 w448 w463 w477 w491 w505 w521 w534 w548 w562 w578 w592 w607 w622 w637 w653 w666 w679 w695 w702 w721 w738 w743 w755 w758 w766 w774 w794 w809] -> w325
          tunnel: w332 -> [w342 w356 w361 w378 w393 w417 w432 w444 w459 w473 w487 w501 w515 w530 w544 w558 w572 w588 w603 w618 w632 w647 w660 w673 w686 w693 w705 w728 w739 w750 w754 w757 w764 w773 w792 w806]
          tunnel: [w341 w356 w362 w382 w396 w409 w424 w438 w452 w465 w480 w494 w507 w520 w537 w550 w565 w579 w596 w611 w625 w640 w651 w664 w677 w691 w705 w720 w734 w742 w754 w757 w764 w773 w792 w806] -> w331
          tunnel: [_ _ _ _ _ _ _ _ _ _ _ _ _ _ _ _ _ _ _ _ _ _ _ _ _ _ _ _ _ _ _ _ _ _ w791 _] -> w330
          tunnel: w328 -> [_ _ w370 w388 w402 w416 w431 w443 w458 w472 w486 w500 w514 w529 w543 w557 w571 w586 w602 w617 w631 w646 w658 w671 w684 _ w712 w726 w737 w748 _ _ _ w772 w790 _]
          tunnel: w327 -> [w343 _ _ _ _ _ _ _ _ _ _ _ _ _ _ _ _ _ _ _ _ _ _ _ _ _ _ _ _ _ _ _ _ w770 w785 _]
          frame "Initialize" {
            w337 = "Initial Message" ("Initial Message")
            # "Initialize - Any operation that needs to be done before the module can receive messages. Synchronize Caller Events.vi will inform Start Module.vi that the module has launched and is ready to receive messages. Module Did Init.vi will broadcast that the module initialized."
            n135 = call "Synchronize Caller Events.vi"("error in"=w353, "Singleton Module Admin in"=w343) -> ("error out"=w352:errorcluster, "Singleton Module Admin out"=w338:refnum<class "Delacor_lib_QMH_Module Admin.lvclass">)  [unwired: 8 in]
            n136 = property on="Property Node" class="Module Admin"(reference=w338) -> ("Accessors:External Launch"=w347:bool)  [unwired: 1 in, 2 out]
            n137 = Select(t=T35."Hidden" ("State"), s=w347, f=T35."Standard" ("State")) -> (s? t:f=w344:T35)
            n138 = call "Module Name--constant.vi"() -> ("Module Name"=w350:string)  [unwired: 11 in]
            n139 = property on="Property Node" class="VI"("Front Panel.Title"=w350) -> (reference out=w349:refnum<vi>, error out=w355:errorcluster)  [unwired: 2 in]
            n140 = invoke on="Invoke Node" class="VI" method="FP.Open"(reference=w349, error in=w355, "State"=w344) -> (reference out=w348:refnum<vi>, error out=w354:errorcluster)  [unwired: 2 in, 3 out]
            n141 = Bundle By Name(cluster=w342, "Status"=w337) -> (w341:T2)
            n142 = invoke on="Invoke Node" class="VI" method="FP.Center"(reference=w348, error in=w354) -> ()  [unwired: 1 in, 3 out]
            n143 = property on="Pane" class="Pane"("Origin"=T34 {"Horizontal"=0, "Vertical"=0}) -> ()  [unwired: 2 in, 2 out]
            n144 = call "Read Config Data.vi"("error in"=w352) -> ("error out"=w335:errorcluster)  [unwired: 10 in]
            n145 = call "Module Name--constant.vi"() -> ("Module Name"=w339:string)  [unwired: 11 in]
            n146 = call "Module Did Init.vi"("error in"=w335, "Initialized?"=TRUE, "Origin"=w339) -> ("error out"=w351:errorcluster)  [unwired: 8 in]
            "Status" <- w337
          }
          frame "---Module Specific---" {
            # "Separator -- The following cases handle messages specific to this Module."
          }
          frame "New VI" {
            # "Creates a new VI in the LabVIEW IDE. The VI Reference is stored and returned. This Reference can later be used to e.g. add modifications to the VI."
            n147 = Variant To Data(error in=w372, type=T6 {"Open Frontpanel"=TRUE, "Wait Notifier"=refnum, "wait for reply"=FALSE} ("New VI Argument"), Variant=w370) -> (data=w368:T6, error out=w371:errorcluster)
            n148 = Unbundle By Name(w368) -> ("Open Frontpanel"=w359:bool, "Wait Notifier"=w367:refnum<notifier>, "wait for reply"=w366:bool)
            n149 = call "Create New VI.vi"("Open Frontpanel"=w359, "Data Cluster in"=w361) -> ("message"=w360:string, "ID"=w358:i32, "Data Cluster out"=w362:T2)  [unwired: 7 in]
            n150 = Bundle By Name(cluster=T36 {"VI Reference"=0, "Result"="", "error"={"status"=FALSE, "code"=0, "source"=""}} ("New VI (Reply Payload)"), "Result"=w360, "VI Reference"=w358) -> (w365:T36)
            n151 = Merge Errors(w371) -> (w363:errorcluster)
            n152 = case "DQMH_FIRE_NOTIFIER" shown="True" w366 {
              tunnel: w367 -> [_ w374]
              tunnel: w365 -> [_ w373]
              frame False {
              }
              frame True {
                n153 = Send Notification(notification=w373, notifier=w374) -> ()  [unwired: 1 in, 2 out]
              }
            }
          }
          frame "Add Object" {
            # "Adds an object to the block diagram or frontpanel of the referenced vi. Get a VI reference from \"New VI\".\nAllowed object names are:\n.NET Container\n.NET Refnum\n2D Picture\n3D Picture\nAbsolute Value\nAccept TLS\nAccess Rights\nActiveX Container\nAdd\nAdd (with error terminals)\nAdd Array Elements\nAdd Entropy\nAdd Private Key To TLS Configuration\nAdd Trusted Certificate To TLS Configuration\nAgitator\nAllSpoll\nAlways Copy\nAnd\nAnd Array Elements\nAppend True/False String\nApplication Refnum\nArray (block diagram constant)\nArray (classic)\nArray (modern)\nArray Interface Control\nArray Max & Min\nArray of Strings to Path\nArray Size\nArray Subset\nArray To Cluster\nArray To Spreadsheet String\nArrayMemInfo\nAssert Structural Type Match\nAssert Structural Type Mismatch\nAtmospheric Tank (classic)\nAtmospheric Tank (modern)\nAutomation Close\nAutomation Open\nAutomation Refnum\nAvogadro Constant (1/mol)\nBase 10 Logarithm Of e\nBin #1\nBin #2\nBitpack to Array\nBluetooth Close Connection\nBluetooth Create Listener\nBluetooth Discover\nBluetooth Network Connection Refnum\nBluetooth Open Connection\nBluetooth Read\nBluetooth Wait On Listener\nBluetooth Write\nBoolean Array To Number\nBoolean To (0,1)\nBuild Array\nBuild Cluster Array\nBuild Map\nBuild Matrix\nBuild Path\nBuild Set\nBuild Waveform\nBundle\nBundle By Name\nByte Array To String\nByte Array To UTF-8 String\nByte Stream File Refnum\nCall By Reference\nCall Chain\nCall Library Function Node\nCall MATLAB Function\nCall Parent Class Method\nCAN Channel (block diagram constant)\nCAN Channel (classic)\nCAN Channel (modern)\nCAN Channel (system)\nCAN Interface (block diagram constant)\nCAN Interface (classic)\nCAN Interface (modern)\nCAN Interface (system)\nCAN Task (block diagram constant)\nCAN Task (classic)\nCAN Task (modern)\nCAN Task (system)\nCancel Button (modern)\nCancel Button (system)\nCancel Notification\nCarriage Return Constant\nCase Structure\nCast Unit Bases\nCheck Valve\nCheckbox (classic)\nCheckBox (modern)\nCheckbox (system)\nClass Specifier Constant\nClassic Color Box\nClassic Color Ramp\nClassic Horizontal Slide Switch\nClassic Vertical Slide\nClear Fixed-Point Overflow Status\nClose File\nClose File (deprecated)\nClose MATLAB Session\nClose Python Session\nClose Reference\nClose TLS Configuration\nClose Variable Connection\nClosure Structure\nCluster (classic)\nCluster (modern)\nCluster Constant\nCluster To Array\nCode Interface Node\nCoerce To Type\nCollection Size\nColor Box Constant\nColor Box Thin Border\nColored Rectangle (broken?)\nCombo Box (classic)\nCombo Box (modern)\nCombo Box (system)\nCombo Box Constant\nComplex Conjugate\nComplex To Polar\nComplex To Re/Im\nCompound Arithmetic\nCompressor\nConcatenate Strings\nConditional Disable Structure\nConstructor Node\nControl & Simulation Loop\nControl Help Window\nControl Online Help\nControl Refnum\nConvert Unit\nConveyer\nCopy\nCopy (deprecated)\nCosecant\nCosine\nCotangent\nCPU Information\nCreate Folder\nCreate Network Stream Endpoint\nCreate Network Stream Reader Endpoint\nCreate Network Stream Writer Endpoint\nCreate Stream\nCreate Unique Network Stream Endpoint\nCreate Unique Network Stream Reader Endpoint\nCreate Unique Network Stream Writer Endpoint\nCreate User Event\nCurrent Processor ID\nCurrent VI's Menubar\nCurrent VI's Path\nDAQmx Analog Trigger Source (block diagram constant)\nDAQmx Analog Trigger Source (classic)\nDAQmx Analog Trigger Source (modern)\nDAQmx Analog Trigger Source (system)\nDAQmx Device Name (block diagram constant)\nDAQmx Device Name (classic)\nDAQmx Device Name (modern)\nDAQmx Device Name (system)\nDAQmx Global Channel (block diagram constant)\nDAQmx Global Channel (classic)\nDAQmx Global Channel (modern)\nDAQmx Global Channel (system)\nDAQmx Physical Channel (block diagram constant)\nDAQmx Physical Channel (classic)\nDAQmx Physical Channel (modern)\nDAQmx Physical Channel (system)\nDAQmx Scale Name (block diagram constant)\nDAQmx Scale Name (classic)\nDAQmx Scale Name (modern)\nDAQmx Scale Name (system)\nDAQmx Switch (block diagram constant)\nDAQmx Switch (classic)\nDAQmx Switch (modern)\nDAQmx Switch (system)\nDAQmx Task Name (block diagram constant)\nDAQmx Task Name (classic)\nDAQmx Task Name (modern)\nDAQmx Task Name (system)\nDAQmx Terminal (block diagram constant)\nDAQmx Terminal (classic)\nDAQmx Terminal (modern)\nDAQmx Terminal (system)\nData Cache Size\nData Log File Refnum\nData Value Reference\nData Value Reference Constant\nDataSocket Close\nDataSocket Open\nDataSocket Read\nDataSocket Refnum\nDataSocket Write\nDate/Time To Seconds\nDecimal Digit?\nDecimal String To Number\nDecimate 1D Array\nDecomposeLockDataValRef\nDecomposeVariant\nDecrement\nDefault Directory\nDelete\nDelete (deprecated)\nDelete Data Value Reference\nDelete From Array\nDelete Menu Items\nDelete Variant Attribute\nDelete Waveform Attribute\nDeny Access\nDequeue Element\nDestroy Stream Endpoint\nDestroy User Event\nDevClear\nDevClearList\nDevice Control/Status\nDevice Refnum\nDiagram Disable Structure\nDial (classic)\nDial (modern)\nDigital Data (classic)\nDigital Data (modern)\nDigital Waveform Graph (classic)\nDigital Waveform Graph (modern)\nDirect Variable Read\nDirect Variable Write\nDivide\nDivide (with error terminals)\nDlg Horiz Scrollbar\nDlg Mac Group Box\nDlg Numeric #1\nDlg Numeric #2\nDlg String\nDlg Vert Scrollbar\nDown Arrow\nDown Bow Valve (flat)\nDown Bow Valve (outline)\nDown Bow Valve (shaded)\nDown Rect Valve (flat)\nDown Rect Valve (outline)\nDown Rect Valve (shaded)\nDown Tee (flat)\nDown Tee (shaded)\nDynamic FPGA Interface Cast\nEased Corner Rectangle\nElement of Set?\nElementary Charge (C)\nEmpty Array?\nEmpty Collection?\nEmpty Path Constant\nEmpty String Constant\nEmpty String/Path?\nEnable Menu Tracking\nEnableLocal\nEnableRemote\nEnd of Line Constant\nEnqueue Element\nEnqueue Element At Opposite End\nEnum (classic)\nEnum (modern)\nEnum (system)\nEnum Constant\nEOF\nEqual To 0?\nEqual?\nError Ring Constant\nEvent Callback Refnum\nEvent Data Node\nEvent Structure\nExchanger\nExclusive Or\nExponential\nExponential (Arg) -1\nExpression Node\nFalse Constant\nFeedback Node\nFieldPoint IO Point (block diagram constant)\nFieldPoint IO Point (classic)\nFieldPoint IO Point (modern)\nFIFO Refnum\nFile Dialog\nFile Dialog (deprecated)\nFile Path Control (classic)\nFile Path Control (modern)\nFile Path Control (system)\nFile Path Indicator (classic)\nFile Path Indicator (modern)\nFile/Directory Info\nFile/Directory Info (deprecated)\nFindLstn\nFindRQS\nFirst Call?\nFixed-Point Overflow?\nFixed-Point to Integer Cast\nFlat Box\nFlat Circle\nFlat Down Triangle\nFlat Frame\nFlat Left Triangle\nFlat Right Triangle\nFlat Round Button\nFlat Rounded Box\nFlat Sequence Structure\nFlat Square Button\nFlat Up Triangle\nFlatten To JSON\nFlatten To String\nFlatten To XML\nFlattened String To Variant\nFloating Point Equal?\nFlush Event Queue\nFlush File\nFlush File (deprecated)\nFlush Queue\nFlush Stream\nFor Loop\nFork\nFormat Date/Time String\nFormat Into File\nFormat Into String\nFormat Value\nFormula Node\nFPGA Refnum to Session\nFract/Exp String To Number\nFramed Color Box (classic)\nFramed Color Box (modern)\nFree Label\nFurnace\nGauge (classic)\nGauge (modern)\nGauge for Simon\nGenerate Front Panel Activity\nGenerate Occurrence\nGenerate User Event\nGenerate User-Defined Trace Event\nGet Control Values by Index\nGet Datalog Position\nGet Date/Time In Seconds\nGet Date/Time String\nGet Drag Drop Data\nGet File Position\nGet File Size\nGet Fixed-Point Components\nGet Help Window Status\nGet Matrix Diagonal\nGet Matrix Elements\nGet Menu Item Info\nGet Menu Selection\nGet Menu Short Cut Info\nGet Notifier Status\nGet Number of Records\nGet Permissions\nGet Queue Status\nGet Submatrix\nGet Type and Creator\nGet Variant Attribute\nGet Volume Info\nGet Waveform Attribute\nGet Waveform Components\nGlobal Variable\nGPIB Clear\nGPIB Initialization\nGPIB Misc\nGPIB Read\nGPIB Serial Poll\nGPIB Status\nGPIB Trigger\nGPIB Wait\nGPIB Write\nGravitational Constant (N m2/kg2)\nGreater Or Equal To 0?\nGreater Or Equal?\nGreater Than 0?\nGreater?\nHandle Peek\nHandle Poke\nHex Digit?\nHexadecimal String To Number\nHopper #1\nHopper #2\nHoriz Line\nHoriz Pipe (flat)\nHoriz Pipe (shaded)\nHorizontal Button Box\nHorizontal Fill Slide (classic)\nHorizontal Fill Slide (modern)\nHorizontal Gradient Oval\nHorizontal Gradient Rectangle\nHorizontal Gradient Rounded Rectangle\nHorizontal Graduated Bar\nHorizontal Pointer Slide (classic)\nHorizontal Pointer Slide (modern)\nHorizontal Pointer Slide (system)\nHorizontal Progress Bar (modern)\nHorizontal Progress Bar (system)\nHorizontal Scrollbar\nHorizontal Slide (classic)\nHorizontal Slide (system)\nHorizontal Smooth Box\nHorizontal Splitter Bar\nHorizontal Splitter Bar (Classic)\nHorizontal Splitter Bar (NXG Style)\nHorizontal Splitter Bar (System)\nHorizontal Switch\nHorizontal Tank\nHorizontal Toggle Switch (classic)\nHorizontal Toggle Switch (modern)\nHyperbolic Cosecant\nHyperbolic Cosine\nHyperbolic Cotangent\nHyperbolic Secant\nHyperbolic Sine\nHyperbolic Tangent\nIMAQ Session\nImplies\nIn Place Element Structure\nIn Range and Coerce\nInclude Fixed-Point Overflow Status\nIncrement\nIndex & Bundle Cluster Array\nIndex Array\nIndex String Array\nInitialize Array\nInline C Node\nInsert Into Array\nInsert Into Map\nInsert Into Set\nInsert Menu Items\nInteger to Fixed-Point Cast\nIntensity Chart (classic)\nIntensity Chart (modern)\nIntensity Graph (classic)\nIntensity Graph (modern)\nInterleave 1D Arrays\nInterpolate 1D Array\nInverse Cosecant\nInverse Cosine\nInverse Cotangent\nInverse Hyperbolic Cosecant\nInverse Hyperbolic Cosine\nInverse Hyperbolic Cotangent\nInverse Hyperbolic Secant\nInverse Hyperbolic Sine\nInverse Hyperbolic Tangent\nInverse Secant\nInverse Sine\nInverse Tangent\nInverse Tangent (2 Input)\nInvoke Node\nIP To String\nIrDA Close Connection\nIrDA Create Listener\nIrDA Discover\nIrDA Network Connection Refnum\nIrDA Open Connection\nIrDA Read\nIrDA Wait On Listener\nIrDA Write\nIsDebuggingActive\nIVI Delete Session\nIVI Logical Name (block diagram constant)\nIVI Logical Name (classic)\nIVI Logical Name (modern)\nIVI New Session\nJoin\nJoin Numbers\nJunction\nKnob (classic)\nKnob (modern)\nLabel (modern)\nLabel (system)\nLabeled Oblong Button\nLabeled Rectangular Button\nLabeled Round Button\nLabeled Square Button\nLabVIEW Object\nLeak Variant Value Reference\nLED Button\nLeft Arrow\nLeft Bow Valve (flat)\nLeft Bow Valve (outline)\nLeft Bow Valve (shaded)\nLeft Down Elbow (flat)\nLeft Down Elbow (shaded)\nLeft Pump (flat)\nLeft Pump (shaded)\nLeft Rect Valve (flat)\nLeft Rect Valve (outline)\nLeft Rect Valve (shaded)\nLeft Tee (flat)\nLeft Tee (shaded)\nLeft Up Elbow (flat)\nLeft Up Elbow (shaded)\nLess Or Equal To 0?\nLess Or Equal?\nLess Than 0?\nLess?\nLexical Class\nLine (chiseled, system)\nLine (chiseled, thick)\nLine (chiseled, thin)\nLine (thick)\nLine (thin)\nLine Feed Constant\nLine with Arrow (thick)\nLine with Arrow (thin)\nList Directory\nList Folder\nListbox (classic)\nListbox (modern)\nListbox (system)\nListbox Symbol Ring Constant\nLoad Certificates Into Memory\nLoad Private Key Into Memory\nLocal Variable\nLock Range\nLogarithm Base 10\nLogarithm Base 2\nLogarithm Base X\nLogical Shift\nLook In Map\nLookup Channel Probe\nLossy Enqueue Element\nLowered Box (thick)\nLowered Rounded Box\nMachine Epsilon\nMake TLS Configuration Immutable\nMakeAddr\nMantissa & Exponent\nMap\nMap Constant\nMatch First String\nMatch Pattern\nMatch True/False String\nMathScript Call By Reference\nMathScript Node\nMATLAB script\nMATLAB Session Refnum\nMatrix Size\nMax & Min\nMenu Refnum\nMenu Ring (classic)\nMenu Ring (modern)\nMenu-Popup Ring\nMerge Errors\nMerge Signals\nMeter (classic)\nMeter (modern)\nMixed Checkbox (system)\nMixed Signal Graph\nMolar Gas Constant (J/(mol K))\nMotion Resource (block diagram constant)\nMotion Resource (classic)\nMotion Resource (modern)\nMotor (flat)\nMotor (shaded)\nMove\nMove (deprecated)\nMulti-Segment Pipe\nMulticolumn Listbox (classic)\nMulticolumn Listbox (modern)\nMulticolumn Listbox (system)\nMultiply\nMultiply (with error terminals)\nMultiply Array Elements\nMultirate Structure\nNatural Logarithm\nNatural Logarithm (Arg +1)\nNatural Logarithm Base\nNatural Logarithm Of 10\nNatural Logarithm Of 2\nNatural Logarithm Of Pi\nNegate\nNegative Infinity\nNew Data Value Reference\nNew Directory\nNew File\nNew TLS Configuration\nNew VI\nNew VI Object\nNot\nNot A Number/Path/Refnum?\nNot A Path Constant\nNot a Refnum Constant\nNot a Shared Variable\nNot And\nNot Equal To 0?\nNot Equal?\nNot Exclusive Or\nNot Or\nNotifier Refnum\nNumber of Cache Levels\nNumber To Boolean Array\nNumber To Decimal String\nNumber To Engineering String\nNumber To Exponential String\nNumber To Fractional String\nNumber To Hexadecimal String\nNumber To Octal String\nNumeric Constant\nNumeric Control (classic)\nNumeric Control (modern)\nNumeric Control (system)\nNumeric Indicator (classic)\nNumeric Indicator (modern)\nObtain Notifier\nObtain Queue\nOccurrence Refnum\nOctal Digit?\nOctal String To Number\nOK Button (modern)\nOK Button (system)\nOld VISA Open\nOLE Variant\nOne Button Dialog\nOpen and Verify Variable Connection\nOpen Application Reference\nOpen Device\nOpen Dynamic Bitfile Reference\nOpen File\nOpen MATLAB Session\nOpen Python Session\nOpen Tank (flat classic)\nOpen Tank (shaded classic)\nOpen Variable Connection\nOpen Variable Connection in Background\nOpen VI Object Reference\nOpen VI Reference\nOpen/Create/Replace Datalog\nOpen/Create/Replace File\nOr\nOr Array Elements\nOval with Shadow\nPackage Matrix\nPassControl\nPath Constant\nPath to Array of Strings\nPath To String\nPath Type\nPi\nPi Divided By 2\nPi Multiplied By 2\nPick Line\nPict Ring (classic)\nPict Ring (modern)\nPict Ring (system)\nPixMap\nPixMap (warning: dangerous)\nPlanck's Constant (J/Hz)\nPlatform Flat Square Button\nPlug-In Control\nPolar To Complex\nPolar To Re/Im\nPositive Infinity\nPower Of 10\nPower Of 2\nPower Of X\nPPoll\nPPollConfig\nPPollUnconfig\nPreallocated Read from Binary File\nPreserve Run-Time Class\nPressure Tank (flat)\nPressure Tank (shaded)\nPreview Queue Element\nPrintable?\nProperty Node\nPulldown Menu Ring\nPush Button\nPython Node\nPython Session Refnum\nQueue Refnum\nQuit LabVIEW\nQuotient & Remainder\nRace Structure\nRadio Button (system)\nRadio Buttons (classic)\nRadio Buttons (modern)\nRadio Buttons (system)\nRaised Box (classic)\nRaised Box (modern)\nRaised Circle\nRaised Down Triangle\nRaised Frame\nRaised Left Triangle\nRaised Right Triangle\nRaised Rounded Box\nRaised Up Triangle\nRandom Number (0-1)\nRcvRespMsg\nRe-accept TLS\nRe/Im To Complex\nRe/Im To Polar\nRead Datalog\nRead Device\nRead File\nRead from Binary File\nRead from Text File\nRead Map Max & Min Keys\nRead Multiple Elements from Stream\nRead Set Max & Min\nRead Single Element from Stream\nRead Variable\nRead Variable with Timeout\nReadStatus\nReceive\nReceiveSetup\nRecessed Box\nRecessed Circle\nRecessed Down Triangle\nRecessed Frame (modern)\nRecessed Frame (system)\nRecessed Left Triangle\nRecessed Menu Ring\nRecessed Right Triangle\nRecessed Rounded Box\nRecessed Up Triangle\nReciprocal\nReciprocal Of e\nReciprocal Of Pi\nRecomposeUnlockDataValRef (warning: dangerous)\nRecomposeVariant (warning: dangerous)\nRectangular Stop Button\nRefnum to Path\nRefnum to Session\nRegion\nRegister Event Callback\nRegister For Events\nRegister Session\nRelease Notifier\nRelease Queue\nRemove Fixed-Point Overflow Status\nRemove From Map\nRemove From Set\nReplace Array Subset\nReplace Substring\nRequest Deallocation\nResetSys\nReshape Array\nResize Matrix\nResource Index\nReverse 1D Array\nReverse String\nRight Arrow\nRight Bow Valve (flat)\nRight Bow Valve (outline)\nRight Bow Valve (shaded)\nRight Down Elbow (flat)\nRight Down Elbow (shaded)\nRight Pump (flat)\nRight Pump (shaded)\nRight Rect Valve (flat)\nRight Rect Valve (outline)\nRight Rect Valve (shaded)\nRight Tee (flat)\nRight Tee (shaded)\nRight Up Elbow (flat)\nRight Up Elbow (shaded)\nRocker\nRotary Feeder\nRotate\nRotate 1D Array\nRotate Left With Carry\nRotate Right With Carry\nRotate String\nRound Button\nRound LED (classic)\nRound LED (modern)\nRound Light\nRound Push Button\nRound Push Button (profile)\nRound Radio Button\nRound Stop Button\nRound To Nearest\nRound Toward +Infinity\nRound Toward -Infinity\nRounded Rectangle with Shadow\nRT FIFO Create\nRT FIFO Delete\nRT FIFO Read\nRT FIFO Write\nRydberg Constant (1/m)\nScale By Power Of 2\nScan From File\nScan From String\nScan String For Tokens\nScan Value\nScanned Variable Read\nScanned Variable Write\nSearch 1D Array\nSearch and Replace String\nSearch Variable Container\nSearch/Split String\nSecant\nSeconds To Date/Time\nSeek\nSelect\nSend\nSend Notification\nSendCmds\nSendDataBytes\nSendIFC\nSendList\nSendLLO\nSendSetup\nSession to Refnum\nSet\nSet Constant\nSet Control Values by Index\nSet Datalog Position\nSet File Position\nSet File Size\nSet Matrix Diagonal\nSet Matrix Elements\nSet Menu Item Info\nSet Number of Records\nSet Occurrence\nSet Permissions\nSet Submatrix\nSet Type and Creator\nSet Variant Attribute\nSet Waveform Attribute\nSetRWLS\nSetTimeOut\nShared Variable\nShared Variable Constant\nShared Variable Control (classic)\nShared Variable Control (modern)\nShared Variable to String\nSign\nSimple Horizontal Slide\nSimple Numeric\nSimple String\nSimple Vertical Slide\nSinc\nSine\nSine & Cosine\nSize Handle\nSlide Switch\nSmoothed Oval\nSmoothed Rounded Rectangle\nSort 1D Array\nSort Array of String\nSpeed Of Light In Vacuum (m/sec)\nSpin Control (system)\nSplit 1D Array\nSplit Button\nSplit Number\nSplit Signals\nSpreadsheet String To Array\nSquare\nSquare Button\nSquare LED (classic)\nSquare LED (modern)\nSquare Light\nSquare Push Button\nSquare Push Button (profile)\nSquare Radio Button\nSquare Root\nStacked Sequence Structure\nStart TLS\nState\nState Diagram\nStatic VI Reference\nStop\nStop Button\nString Constant\nString Control (classic)\nString Control (modern)\nString Control (system)\nString Indicator (classic)\nString Indicator (modern)\nString Length\nString Subset\nString To Byte Array\nString To IP\nString To Path\nString to Shared Variable\nStrip Path\nSubPanel\nSubPanel (Classic)\nSubPanel (NXG Style)\nSubPanel (System)\nSubtract\nSubtract (with error terminals)\nSwap Bytes\nSwap Values\nSwap Vector Element\nSwap Words\nTab Constant\nTab Control (classic)\nTab Control (modern)\nTab Control (NXG Style)\nTab Control (system)\nTable (classic)\nTable (modern)\nTable (system)\nTag Attribute Ring\nTangent\nTank (classic)\nTank (modern)\nTarget Structure\nTCP Close Connection\nTCP Create Listener\nTCP Flattened Read\nTCP Flattened Write\nTCP Flex Read\nTCP Flex Write\nTCP Network Connection Refnum\nTCP Open Connection\nTCP Read\nTCP Wait On Listener\nTCP Write\nTDMS Advanced Asynchronous Read (Data Ref)\nTDMS Advanced Asynchronous Write (Data Ref)\nTDMS Close\nTDMS Configure Asynchronous Reads (Data Ref)\nTDMS Configure Asynchronous Writes (Data Ref)\nTDMS Defragment\nTDMS Delete Data\nTDMS File\nTDMS Flush\nTDMS Get Asynchronous Read Status (Data Ref)\nTDMS Get Asynchronous Write Status (Data Ref)\nTDMS Get Properties\nTDMS In Memory Close\nTDMS In Memory Open\nTDMS In Memory Read Bytes\nTDMS List Contents\nTDMS Open\nTDMS Read\nTDMS Refnum To File ID\nTDMS Set Properties\nTDMS Write\nTDMS Write IP\nTemporary Directory\nTestSRQ\nTestSys\nText & Pict Ring (classic)\nText & Pict Ring (modern)\nText Button\nText Ring (block diagram constant)\nText Ring (classic)\nText Ring (modern)\nText Ring (system)\nText to UTF-8\nThermometer (classic)\nThermometer (modern)\nThreshold 1D Array\nTick Count (ms)\nTime Stamp (block diagram constant)\nTime Stamp Control (classic)\nTime Stamp Control (modern)\nTime Stamp Control (system)\nTime Stamp Indicator (classic)\nTime Stamp Indicator (modern)\nTimed Loop\nTimed Sequence\nTLS configuration\nTLS Connection?\nTo Byte Integer\nTo Double Precision Complex\nTo Double Precision Float\nTo Extended Precision Complex\nTo Extended Precision Float\nTo Fixed-Point\nTo Long Integer\nTo Lower Case\nTo More Generic Class\nTo More Specific Class\nTo OLE Variant\nTo Probe String\nTo Quad Integer\nTo Single Precision Complex\nTo Single Precision Float\nTo Time Stamp\nTo Unsigned Byte Integer\nTo Unsigned Long Integer\nTo Unsigned Quad Integer\nTo Unsigned Word Integer\nTo Upper Case\nTo Variant\nTo Word Integer\nTraditional DAQ Channel (block diagram constant)\nTraditional DAQ Channel (classic)\nTraditional DAQ Channel (modern)\nTranspose 1D Array\nTranspose 2D Array\nTranspose Matrix\nTree (classic)\nTree (modern)\nTree (system)\nTrigger\nTriggerList\nTwo Button Dialog\nType and Creator\nType Cast\nType Error\nType Must Be Array\nType Must Be Cluster\nType Of\nType Specialization Structure\nUDP Close\nUDP Multicast Open\nUDP Network Connection Refnum\nUDP Open\nUDP Read\nUDP Write\nUnbitpack from Array\nUnbundle\nUnbundle By Name\nUnflatten From JSON\nUnflatten From String\nUnflatten From XML\nUnleak Variant Value Reference\nUnpackage Matrix\nUnregister For Events\nUnregister Session\nUp Arrow\nUp Bow Valve (flat)\nUp Bow Valve (outline)\nUp Bow Valve (shaded)\nUp Rect Valve (flat)\nUp Rect Valve (outline)\nUp Rect Valve (shaded)\nUp Tee (flat)\nUp Tee (shaded)\nUser Defined Refnum\nUser Defined Refnum Tag (block diagram constant)\nUser Defined Refnum Tag (classic)\nUser Defined Refnum Tag (modern)\nUser Defined Refnum Tag Flatten (classic)\nUser Defined Refnum Tag Flatten (modern)\nUser Defined Tag (block diagram constant)\nUser Defined Tag (classic)\nUser Defined Tag (modern)\nUser Item\nUTF-8 String To Byte Array\nUTF-8 to Text\nVariable Class Specifier Constant\nVariable Name Constant\nVariant\nVariant To Data\nVariant To Flattened String\nVert Line\nVert Pipe (flat)\nVert Pipe (shaded)\nVert Rocker\nVertical Fill Slide (classic)\nVertical Fill Slide (modern)\nVertical Gradient Oval\nVertical Gradient Rectangle\nVertical Gradient Rounded Rectangle\nVertical Graduated Bar\nVertical Pointer Slide (classic)\nVertical Pointer Slide (modern)\nVertical Pointer Slide (system)\nVertical Progress Bar (modern)\nVertical Progress Bar (system)\nVertical Scrollbar\nVertical Slide (system)\nVertical Slide Switch (classic)\nVertical Slide Switch (modern)\nVertical Smooth Box\nVertical Splitter Bar\nVertical Splitter Bar (Classic)\nVertical Splitter Bar (NXG Style)\nVertical Splitter Bar (System)\nVertical Switch\nVertical Toggle Switch (classic)\nVertical Toggle Switch (modern)\nVI Library\nVI Refnum\nVI Server Reference\nVISA Assert Interrupt Signal\nVISA Assert Trigger\nVISA Assert Utility Signal\nVISA Clear\nVISA Close\nVISA Disable Event\nVISA Discard Events\nVISA Enable Event\nVISA Find Resource\nVISA Flush I/O Buffer\nVISA GPIB Command\nVISA GPIB Control ATN\nVISA GPIB Control REN\nVISA GPIB Pass Control\nVISA GPIB Send IFC\nVISA In 16\nVISA In 32\nVISA In 64\nVISA In 8\nVISA Lock\nVISA Map Address\nVISA Map Trigger\nVISA Memory Allocation\nVISA Memory Allocation Ex\nVISA Memory Free\nVISA Move\nVISA Move In 16\nVISA Move In 32\nVISA Move In 64\nVISA Move In 8\nVISA Move Out 16\nVISA Move Out 32\nVISA Move Out 64\nVISA Move Out 8\nVISA Open\nVISA Out 16\nVISA Out 32\nVISA Out 64\nVISA Out 8\nVISA Peek 16\nVISA Peek 32\nVISA Peek 64\nVISA Peek 8\nVISA Poke 16\nVISA Poke 32\nVISA Poke 64\nVISA Poke 8\nVISA Read\nVISA Read STB\nVISA Read To File\nVISA Refnum to Session\nVISA Resource Name\nVISA resource name (classic)\nVISA resource name (modern)\nVISA Set I/O Buffer Size\nVISA Status Description\nVISA Unlock\nVISA Unmap Address\nVISA Unmap Trigger\nVISA USB Control In\nVISA USB Control Out\nVISA VXI Cmd or Query\nVISA Wait on Event\nVISA Write\nVISA Write From File\nVolume Info\nWait (ms)\nWait For Activity\nWait For Front Panel Activity\nWait for GPIB RQS\nWait on Notification\nWait on Notification from Multiple\nWait on Notification from Multiple with Notifier History\nWait on Notification with Notifier History\nWait on Occurrence\nWait Until Next ms Multiple\nWaitSRQ\nWaveform Chart\nWaveform Chart (classic)\nWaveform Chart (modern)\nWaveform Graph (classic)\nWaveform Graph (modern)\nWhile Loop #1\nWhile Loop #2\nWhite Space?\nWrite Datalog\nWrite Device\nWrite File\nWrite Multiple Elements to Stream\nWrite Single Element to Stream\nWrite to Binary File\nWrite to Text File\nWrite Variable\nWrite Variable with Timeout\nXY Graph (classic)\nXY Graph (modern)\nY-th Root of X"
            n154 = Variant To Data(error in=w389, type=T7 {"VI Reference"=0, "Object Name"="", "Wait Notifier"=refnum, "wait for reply"=FALSE, "position_x"=0, "position_y"=0} ("Add Object Argument"), Variant=w388) -> (data=w375:T7, error out=w377:errorcluster)
            n155 = Unbundle By Name(w375) -> ("Wait Notifier"=w386:refnum<notifier>, "wait for reply"=w385:bool)
            n156 = control-ref of="Ring 2"() -> (w379:refnum<vi>)
            n157 = call "add vi object.vi"("Ring in"=w379, "error in (no error)"=w377, "Add Object Argument"=w375, "Data Cluster in"=w378) -> ("error out"=w381:errorcluster, "Result"=w380:string, "object_id"=w376:i32, "Data Cluster out"=w382:T2)  [unwired: 4 in]
            n158 = Bundle By Name(cluster=T37 {"error"={"status"=FALSE, "code"=0, "source"=""}, "Object ID"=0, "Result"=""} ("Add Object (Reply Payload)"), "error"=w381, "Result"=w380, "Object ID"=w376) -> (w384:T37)
            n159 = case "DQMH_FIRE_NOTIFIER" shown="True" w385 {
              tunnel: w386 -> [_ w391]
              tunnel: w384 -> [_ w390]
              frame False {
              }
              frame True {
                n160 = Send Notification(notification=w390, notifier=w391) -> ()  [unwired: 1 in, 2 out]
              }
            }
          }
          frame "Connect Objects" {
            # "Connects two terminals of two objects with a wire on the block diagram of a labview vi. To get a new VI use \"new vi\" to add objects to a vi use \"add object\"."
            n161 = Variant To Data(error in=w403, type=T8 {"vi reference"=0, "from object reference"=0, "to object reference"=0, "from object terminal index"=0, "to object terminal index"=0, "Wait Notifier"=refnum, "wait for reply"=FALSE} ("Connect Objects Argument"), Variant=w402) -> (data=w394:T8, error out=w392:errorcluster)
            n162 = Unbundle By Name(w394) -> ("Wait Notifier"=w400:refnum<notifier>, "wait for reply"=w399:bool)
            n163 = call "Wire Two Objects.vi"("error in (no error)"=w392, "input cluster"=w394, "Data Cluster in"=w393) -> ("error out"=w395:errorcluster, "Data Cluster out"=w396:T2)  [unwired: 7 in]
            n164 = Bundle By Name(cluster=T38 {"result"="", "error"={"status"=FALSE, "code"=0, "source"=""}} ("Connect Objects (Reply Payload)"), "error"=w395) -> (w398:T38)
            n165 = case "DQMH_FIRE_NOTIFIER" shown="True" w399 {
              tunnel: w400 -> [_ w405]
              tunnel: w398 -> [_ w404]
              frame False {
              }
              frame True {
                n166 = Send Notification(notification=w404, notifier=w405) -> ()  [unwired: 1 in, 2 out]
              }
            }
          }
          frame "Get Object Terminals" {
            # "Returns the Terminals Names and/or descriptions as a string as well as their Index to be used in other functions like connect objects."
            n167 = Variant To Data(error in=w418, type=T9 {"object id"=0, "Wait Notifier"=refnum, "wait for reply"=FALSE} ("Get Object Terminals Argument"), Variant=w416) -> (data=w410:T9, error out=w406:errorcluster)
            n168 = Unbundle By Name(w410) -> ("Wait Notifier"=w414:refnum<notifier>, "wait for reply"=w413:bool)
            n169 = call "get terminal info.vi"("error in (no error)"=w406, "Get Object Terminals Argument"=w410, "Data Cluster in"=w417) -> ("error out"=w408:errorcluster, "String"=w407:string, "Data Cluster out"=w409:T2)  [unwired: 6 in]
            n170 = Bundle By Name(cluster=T39 {"terminals description"="", "error"={"status"=FALSE, "code"=0, "source"=""}} ("Get Object Terminals (Reply Payload)"), "terminals description"=w407, "error"=w408) -> (w412:T39)
            n171 = case "DQMH_FIRE_NOTIFIER" shown="True" w413 {
              tunnel: w414 -> [_ w420]
              tunnel: w412 -> [_ w419]
              frame False {
              }
              frame True {
                n172 = Send Notification(notification=w419, notifier=w420) -> ()  [unwired: 1 in, 2 out]
              }
            }
          }
          frame "get vi error list" {
            # "Returns the current error list (list you see when clicking the run arrow) in a text format giving information about what on the block diagram needs to be fixed. Use this to see if your actions worked."
            n173 = Variant To Data(error in=w433, type=T10 {"vi id"=0, "Wait Notifier"=refnum, "wait for reply"=FALSE} ("get vi error list Argument"), Variant=w431) -> (data=w425:T10, error out=w421:errorcluster)
            n174 = Unbundle By Name(w425) -> ("Wait Notifier"=w429:refnum<notifier>, "wait for reply"=w428:bool)  [unwired: 1 out]
            n175 = call "generate vi error list.vi"("error in (no error)"=w421, "get vi error list Argument"=w425, "Data Cluster in"=w432) -> ("error out"=w422:errorcluster, "Error Description"=w423:string, "Data Cluster out"=w424:T2)  [unwired: 6 in]
            n176 = Bundle By Name(cluster=T40 {"error list"="", "error"={"status"=FALSE, "code"=0, "source"=""}} ("get vi error list (Reply Payload)"), "error list"=w423, "error"=w422) -> (w427:T40)
            n177 = case "DQMH_FIRE_NOTIFIER" shown="True" w428 {
              tunnel: w429 -> [_ w435]
              tunnel: w427 -> [_ w434]
              frame False {
              }
              frame True {
                n178 = Send Notification(notification=w434, notifier=w435) -> ()  [unwired: 1 in, 2 out]
              }
            }
          }
          frame "Cleanup VI" {
            # "Cleans up the block diagram of a vi referenced by reference number."
            n179 = Variant To Data(error in=w445, type=T11 {"vi reference"=0, "Wait Notifier"=refnum, "wait for reply"=FALSE} ("Cleanup VI Argument"), Variant=w443) -> (data=w437:T11, error out=w436:errorcluster)
            n180 = Unbundle By Name(w437) -> ("Wait Notifier"=w441:refnum<notifier>, "wait for reply"=w440:bool)
            n181 = call "clean up vis blockdiagram.vi"("error in (no error)"=w436, "Cleanup VI Argument"=w437, "Data Cluster in"=w444) -> ("Cleanup VI (Reply Payload)"=w439:T56, "Data Cluster out"=w438:T2)  [unwired: 6 in, 1 out]
            n182 = case "DQMH_FIRE_NOTIFIER" shown="True" w440 {
              tunnel: w441 -> [_ w447]
              tunnel: w439 -> [_ w446]
              frame False {
              }
              frame True {
                n183 = Send Notification(notification=w446, notifier=w447) -> ()  [unwired: 1 in, 2 out]
              }
            }
          }
          frame "create_control" {
            # "Creates a control or indicator on the terminal specified by Object ID and Terminal Index, depending on if it's a in- or output of the node. If Constant is set to True, it can only be used on node inputs and will create a constant.\nIt will return the reference to the created control or indicator, that is a reference to the frontpanel element. If constant is True it returns a reference to the block diagram object (constant)."
            n184 = Variant To Data(error in=w460, type=T12 {"Object ID"=0, "Terminal Index"=0, "Constant"=FALSE, "Wait Notifier"=refnum, "wait for reply"=FALSE, "Value"=""} ("create_control Argument"), Variant=w458) -> (data=w451:T12, error out=w448:errorcluster)
            n185 = Unbundle By Name(w451) -> ("Wait Notifier"=w456:refnum<notifier>, "wait for reply"=w455:bool)  [unwired: 3 out]
            n186 = call "Do Create Control.vi"("error in (no error)"=w448, "create_control Argument"=w451, "Data Cluster in"=w459) -> ("error out"=w449:errorcluster, "new reference"=w450:i32, "Data Cluster out"=w452:T2)  [unwired: 6 in]
            n187 = Bundle By Name(cluster=T41 {"Object ID"=0, "error"={"status"=FALSE, "code"=0, "source"=""}} ("create_control (Reply Payload)"), "Object ID"=w450, "error"=w449) -> (w454:T41)
            n188 = case "DQMH_FIRE_NOTIFIER" shown="True" w455 {
              tunnel: w456 -> [_ w462]
              tunnel: w454 -> [_ w461]
              frame False {
              }
              frame True {
                n189 = Send Notification(notification=w461, notifier=w462) -> ()  [unwired: 1 in, 2 out]
              }
            }
          }
          frame "Run VI" {
            # "Runs a VI specified by VI ID and brings the frontpanel to foreground if open_frontpanel is set to True."
            n190 = Variant To Data(error in=w474, type=T13 {"VI ID"=0, "open_frontpanel"=FALSE, "Wait Notifier"=refnum, "wait for reply"=FALSE} ("Run VI Argument"), Variant=w472) -> (data=w466:T13, error out=w463:errorcluster)
            n191 = Unbundle By Name(w466) -> ("Wait Notifier"=w470:refnum<notifier>, "wait for reply"=w469:bool)
            n192 = call "Do Run VI.vi"("error in (no error)"=w463, "Run VI Argument"=w466, "Data Cluster in"=w473) -> ("error out"=w464:errorcluster, "Data Cluster out"=w465:T2)  [unwired: 7 in]
            n193 = Bundle By Name(cluster=T42 {"error"={"status"=FALSE, "code"=0, "source"=""}} ("Run VI (Reply Payload)"), "error"=w464) -> (w468:T42)
            n194 = case "DQMH_FIRE_NOTIFIER" shown="True" w469 {
              tunnel: w470 -> [_ w476]
              tunnel: w468 -> [_ w475]
              frame False {
              }
              frame True {
                n195 = Send Notification(notification=w475, notifier=w476) -> ()  [unwired: 1 in, 2 out]
              }
            }
          }
          frame "add_to_selection" {
            # "Adds an object specified by object_id to the selection list. Use this to copy & paste or enclose a selection. Use clear_selection or remove_from_selection to remove the object from the list. Make sure to check if the selection list looks good."
            n196 = Variant To Data(error in=w488, type=T14 {"object_id"=0, "Wait Notifier"=refnum, "wait for reply"=FALSE, "vi_id"=0} ("add_to_selection Argument"), Variant=w486) -> (data=w479:T14, error out=w477:errorcluster)
            n197 = Unbundle By Name(w479) -> ("Wait Notifier"=w484:refnum<notifier>, "wait for reply"=w483:bool)
            n198 = call "Do Add To Selection.vi"("error in (no error)"=w477, "add_to_selection Argument"=w479, "Data Cluster in"=w487) -> ("error out"=w478:errorcluster, "Data Cluster out"=w480:T2)  [unwired: 7 in]
            n199 = Bundle By Name(cluster=T43 {"Current Selection"=[], "error"={"status"=FALSE, "code"=0, "source"=""}} ("add_to_selection (Reply Payload)"), "error"=w478) -> (w482:T43)
            n200 = case "DQMH_FIRE_NOTIFIER" shown="True" w483 {
              tunnel: w484 -> [_ w490]
              tunnel: w482 -> [_ w489]
              frame False {
              }
              frame True {
                n201 = Send Notification(notification=w489, notifier=w490) -> ()  [unwired: 1 in, 2 out]
              }
            }
          }
          frame "clear_selection_list" {
            # "Clears all elements in the selection list. Use this before making a new selection."
            n202 = Variant To Data(error in=w502, type=T15 {"Wait Notifier"=refnum, "wait for reply"=FALSE, "vi_id"=0} ("clear_selection_list Argument"), Variant=w500) -> (data=w493:T15, error out=w491:errorcluster)
            n203 = Unbundle By Name(w493) -> ("Wait Notifier"=w498:refnum<notifier>, "wait for reply"=w497:bool)
            n204 = call "Do Clear Selection List.vi"("error in (no error)"=w491, "input cluster"=w493, "Data Cluster in"=w501) -> ("error out"=w492:errorcluster, "Data Cluster out"=w494:T2)  [unwired: 7 in]
            n205 = Bundle By Name(cluster=T44 {"error"={"status"=FALSE, "code"=0, "source"=""}} ("clear_selection_list (Reply Payload)"), "error"=w492) -> (w496:T44)
            n206 = case "DQMH_FIRE_NOTIFIER" shown="True" w497 {
              tunnel: w498 -> [_ w504]
              tunnel: w496 -> [_ w503]
              frame False {
              }
              frame True {
                n207 = Send Notification(notification=w503, notifier=w504) -> ()  [unwired: 1 in, 2 out]
              }
            }
          }
          frame "remove_from_selection" {
            # "Removes the object specified by object_id from the current selection list and returns the resulting new list."
            n208 = Variant To Data(error in=w516, type=T16 {"vi_id"=0, "object_id"=0, "Wait Notifier"=refnum, "wait for reply"=FALSE} ("remove_from_selection Argument"), Variant=w514) -> (data=w508:T16, error out=w505:errorcluster)
            n209 = Unbundle By Name(w508) -> ("Wait Notifier"=w512:refnum<notifier>, "wait for reply"=w511:bool)
            n210 = call "Do Remove From Selection.vi"("error in (no error)"=w505, "remove_from_selection Argument"=w508, "Data Cluster in"=w515) -> ("error out"=w506:errorcluster, "Data Cluster out"=w507:T2)  [unwired: 7 in]
            n211 = Bundle By Name(cluster=T45 {"current_selection"=[], "error"={"status"=FALSE, "code"=0, "source"=""}} ("remove_from_selection (Reply Payload)"), "error"=w506) -> (w510:T45)
            n212 = case "DQMH_FIRE_NOTIFIER" shown="True" w511 {
              tunnel: w512 -> [_ w518]
              tunnel: w510 -> [_ w517]
              frame False {
              }
              frame True {
                n213 = Send Notification(notification=w517, notifier=w518) -> ()  [unwired: 1 in, 2 out]
              }
            }
          }
          frame "enclose_selection" {
            # "Use this function to efficiently generate Loops or other structures around existing code. This is the quickest way to create loops including tunnles and wiring, wire the objects first, then create a loop around them, tunnles will be there automatically. Use the add_to_selection, remove_from_selection and clear_selection_list tools to change the current selection, connect_objects to connect them, then call this tool to create a structure around them.\nAllowed values for structure_type are:\nWhile Loop\nFor Loop\nCase Structure\nSequence Structure\nEvent Structure"
            n214 = Variant To Data(error in=w531, type=T17 {"vi_id"=0, "structure_type"="", "Wait Notifier"=refnum, "wait for reply"=FALSE} ("enclose_selection Argument"), Variant=w529) -> (data=w519:T17, error out=w521:errorcluster)
            n215 = Unbundle By Name(w519) -> ("Wait Notifier"=w527:refnum<notifier>, "wait for reply"=w526:bool)  [unwired: 2 out]
            n216 = call "Do Enclose Selection.vi"("error in (no error)"=w521, "enclose_selection Argument"=w519, "Data Cluster in"=w530) -> ("error out"=w522:errorcluster, "object_id"=w523:i32, "Data Cluster out"=w520:T2)  [unwired: 6 in]
            n217 = Bundle By Name(cluster=T46 {"object_id"=0, "error"={"status"=FALSE, "code"=0, "source"=""}} ("enclose_selection (Reply Payload)"), "object_id"=w523, "error"=w522) -> (w525:T46)
            n218 = case "DQMH_FIRE_NOTIFIER" shown="True" w526 {
              tunnel: w527 -> [_ w533]
              tunnel: w525 -> [_ w532]
              frame False {
              }
              frame True {
                n219 = Send Notification(notification=w532, notifier=w533) -> ()  [unwired: 1 in, 2 out]
              }
            }
          }
          frame "rename_object" {
            # "Use this to change an objects Label.Text property. Usually used for frontpanel objects. Use the label_visible True/False to decide if the label is displayed afterwards."
            n220 = Variant To Data(error in=w545, type=T18 {"new_label_name"="", "label_visible"=FALSE, "Wait Notifier"=refnum, "wait for reply"=FALSE, "object_id"=0} ("rename_object Argument"), Variant=w543) -> (data=w536:T18, error out=w534:errorcluster)
            n221 = Unbundle By Name(w536) -> ("Wait Notifier"=w541:refnum<notifier>, "wait for reply"=w540:bool)
            n222 = call "Do Rename Object.vi"("error in (no error)"=w534, "rename_object Argument"=w536, "Data Cluster in"=w544) -> ("error out"=w535:errorcluster, "Data Cluster out"=w537:T2)  [unwired: 7 in]
            n223 = Bundle By Name(cluster=T47 {"error"={"status"=FALSE, "code"=0, "source"=""}} ("rename_object (Reply Payload)"), "error"=w535) -> (w539:T47)
            n224 = case "DQMH_FIRE_NOTIFIER" shown="True" w540 {
              tunnel: w541 -> [_ w547]
              tunnel: w539 -> [_ w546]
              frame False {
              }
              frame True {
                n225 = Send Notification(notification=w546, notifier=w547) -> ()  [unwired: 1 in, 2 out]
              }
            }
          }
          frame "set_value" {
            # "Sets the value of a constant or control/indicator. The value is transferred as a string, but can be also a number."
            n226 = Variant To Data(error in=w559, type=T19 {"object_id"=0, "value"="", "Wait Notifier"=refnum, "wait for reply"=FALSE} ("set_value Argument"), Variant=w557) -> (data=w551:T19, error out=w548:errorcluster)
            n227 = Unbundle By Name(w551) -> ("Wait Notifier"=w555:refnum<notifier>, "wait for reply"=w554:bool)
            n228 = call "Do Set Value.vi"("error in (no error)"=w548, "set_value Argument"=w551, "Data Cluster in"=w558) -> ("error out"=w549:errorcluster, "Data Cluster out"=w550:T2)  [unwired: 7 in]
            n229 = Bundle By Name(cluster=T48 {"error"={"status"=FALSE, "code"=0, "source"=""}} ("set_value (Reply Payload)"), "error"=w549) -> (w553:T48)
            n230 = case "DQMH_FIRE_NOTIFIER" shown="True" w554 {
              tunnel: w555 -> [_ w561]
              tunnel: w553 -> [_ w560]
              frame False {
              }
              frame True {
                n231 = Send Notification(notification=w560, notifier=w561) -> ()  [unwired: 1 in, 2 out]
              }
            }
          }
          frame "delete_object" {
            # "removes the object from the blockdiagram or frontpanel."
            n232 = Variant To Data(error in=w573, type=T20 {"object_id"=0, "Wait Notifier"=refnum, "wait for reply"=FALSE} ("delete_object Argument"), Variant=w571) -> (data=w564:T20, error out=w562:errorcluster)
            n233 = Unbundle By Name(w564) -> ("Wait Notifier"=w569:refnum<notifier>, "wait for reply"=w568:bool)
            n234 = call "Do Delete Object.vi"("error in (no error)"=w562, "delete_object Argument"=w564, "Data Cluster in"=w572) -> ("error out"=w563:errorcluster, "Data Cluster out"=w565:T2)  [unwired: 7 in]
            n235 = Bundle By Name(cluster=T49 {"error"={"status"=FALSE, "code"=0, "source"=""}} ("delete_object (Reply Payload)"), "error"=w563) -> (w567:T49)
            n236 = case "DQMH_FIRE_NOTIFIER" shown="True" w568 {
              tunnel: w569 -> [_ w575]
              tunnel: w567 -> [_ w574]
              frame False {
              }
              frame True {
                n237 = Send Notification(notification=w574, notifier=w575) -> ()  [unwired: 1 in, 2 out]
              }
            }
          }
          frame "save_vi" {
            # "Saves a VI to the specified path. If Path is empty and vi was saved before, it saves to same location"
            n238 = Variant To Data(error in=w589, type=T21 {"vi_id"=0, "path"="", "Wait Notifier"=refnum, "wait for reply"=FALSE} ("save_vi Argument"), Variant=w586) -> (data=w580:T21, error out=w587:errorcluster)
            n239 = Unbundle By Name(w580) -> ("Wait Notifier"=w584:refnum<notifier>, "wait for reply"=w583:bool)
            n240 = call "Do Save VI.vi"("error in (no error)"=w587, "save_vi Argument"=w580, "Data Cluster in"=w588) -> ("error out"=w578:errorcluster, "VI Path"=w577:path, "Data Cluster out"=w579:T2)  [unwired: 6 in]
            n241 = Path To String(path=w577) -> (string=w576:string)
            n242 = Bundle By Name(cluster=T50 {"path_out"="", "error"={"status"=FALSE, "code"=0, "source"=""}} ("save_vi (Reply Payload)"), "path_out"=w576, "error"=w578) -> (w582:T50)
            n243 = case "DQMH_FIRE_NOTIFIER" shown="True" w583 {
              tunnel: w584 -> [_ w591]
              tunnel: w582 -> [_ w590]
              frame False {
              }
              frame True {
                n244 = Send Notification(notification=w590, notifier=w591) -> ()  [unwired: 1 in, 2 out]
              }
            }
          }
          frame "get_structure_diagram" {
            # "Returns the id of a sub-diagram of a structure (the inside of a loop or case-structure). Use this to add objects to a structure instead of to the top level blockdiagram. For Case-Structures, use the index option to iterate through them, for loops ignore index. Also consider using the \"enclose_selection\" tool if you work with structures to make wiring easier."
            n245 = Variant To Data(error in=w604, type=T22 {"structure_id"=0, "index"=0, "Wait Notifier"=refnum, "wait for reply"=FALSE} ("get_structure_diagram Argument"), Variant=w602) -> (data=w595:T22, error out=w592:errorcluster)
            n246 = Unbundle By Name(w595) -> ("Wait Notifier"=w600:refnum<notifier>, "wait for reply"=w599:bool)  [unwired: 2 out]
            n247 = call "Do Get Structure Diagram.vi"("error in (no error)"=w592, "get_structure_diagram Argument"=w595, "Data Cluster in"=w603) -> ("error out"=w593:errorcluster, "diagram_id"=w594:i32, "Data Cluster out"=w596:T2)  [unwired: 6 in]
            n248 = Bundle By Name(cluster=T51 {"diagram_id"=0, "error"={"status"=FALSE, "code"=0, "source"=""}} ("get_structure_diagram (Reply Payload)"), "diagram_id"=w594, "error"=w593) -> (w598:T51)
            n249 = case "DQMH_FIRE_NOTIFIER" shown="True" w599 {
              tunnel: w600 -> [_ w606]
              tunnel: w598 -> [_ w605]
              frame False {
              }
              frame True {
                n250 = Send Notification(notification=w605, notifier=w606) -> ()  [unwired: 1 in, 2 out]
              }
            }
          }
          frame "add_subvi" {
            # "Adds a SubVI to a blockdiagram or sturcture subdiagram similar to the add_object method."
            n251 = Variant To Data(error in=w619, type=T23 {"diagram_id"=0, "subvi_path"="", "Wait Notifier"=refnum, "wait for reply"=FALSE, "position_x"=0, "position_y"=0} ("add_subvi Argument"), Variant=w617) -> (data=w610:T23, error out=w607:errorcluster)
            n252 = Unbundle By Name(w610) -> ("Wait Notifier"=w615:refnum<notifier>, "wait for reply"=w614:bool)  [unwired: 2 out]
            n253 = call "Do Add Subvi.vi"("error in (no error)"=w607, "add_subvi Argument"=w610, "Data Cluster in"=w618) -> ("error out"=w608:errorcluster, "object_id"=w609:i32, "Data Cluster out"=w611:T2)  [unwired: 6 in]
            n254 = Bundle By Name(cluster=T52 {"subvi_id"=0, "error"={"status"=FALSE, "code"=0, "source"=""}} ("add_subvi (Reply Payload)"), "subvi_id"=w609, "error"=w608) -> (w613:T52)
            n255 = case "DQMH_FIRE_NOTIFIER" shown="True" w614 {
              tunnel: w615 -> [_ w621]
              tunnel: w613 -> [_ w620]
              frame False {
              }
              frame True {
                n256 = Send Notification(notification=w620, notifier=w621) -> ()  [unwired: 1 in, 2 out]
              }
            }
          }
          frame "connect_to_pane" {
            # "takes a control_id and connects the corresponding frontpanel control or indicator to the connector pane of the subvi. Do this to all necessary fronpanel controls/indicators to use the VI as a SubVI. The subvis by default have 4 fields on the left and right, and two on top/bottom. Their index starts at the bottom right, and goes counter clockwise."
            n257 = Variant To Data(error in=w633, type=T24 {"control_id"=0, "connector_pane_index"=0, "Wait Notifier"=refnum, "wait for reply"=FALSE} ("connect_to_pane Argument"), Variant=w631) -> (data=w624:T24, error out=w622:errorcluster)
            n258 = Unbundle By Name(w624) -> ("Wait Notifier"=w629:refnum<notifier>, "wait for reply"=w628:bool)  [unwired: 2 out]
            n259 = call "do connect to pane.vi"("error in (no error)"=w622, "connect_to_pane Argument"=w624, "Data Cluster in"=w632) -> ("error out"=w623:errorcluster, "Data Cluster out"=w625:T2)  [unwired: 7 in]
            n260 = Bundle By Name(cluster=T53 {"error"={"status"=FALSE, "code"=0, "source"=""}} ("connect_to_pane (Reply Payload)"), "error"=w623) -> (w627:T53)
            n261 = case "DQMH_FIRE_NOTIFIER" shown="True" w628 {
              tunnel: w629 -> [_ w635]
              tunnel: w627 -> [_ w634]
              frame False {
              }
              frame True {
                n262 = Send Notification(notification=w634, notifier=w635) -> ()  [unwired: 1 in, 2 out]
              }
            }
          }
          frame "get_object_help" {
            # "returns the labview detailed help article including termina descriptions. To get the exact indexes of the terminals use the get terminal info."
            n263 = Variant To Data(error in=w648, type=T25 {"object_id"=0, "Wait Notifier"=refnum, "wait for reply"=FALSE} ("get_object_help Argument"), Variant=w646) -> (data=w639:T25, error out=w637:errorcluster)
            n264 = Unbundle By Name(w639) -> ("Wait Notifier"=w644:refnum<notifier>, "wait for reply"=w643:bool)  [unwired: 1 out]
            n265 = call "Do Get Object Help.vi"("error in (no error)"=w637, "get_object_help Argument"=w639, "Data Cluster in"=w647) -> ("error out"=w636:errorcluster, "help_string"=w638:string, "Data Cluster out"=w640:T2)  [unwired: 6 in]
            n266 = Bundle By Name(cluster=T54 {"help_string"="", "error"={"status"=FALSE, "code"=0, "source"=""}} ("get_object_help (Reply Payload)"), "help_string"=w638, "error"=w636) -> (w642:T54)
            n267 = case "DQMH_FIRE_NOTIFIER" shown="True" w643 {
              tunnel: w644 -> [_ w650]
              tunnel: w642 -> [_ w649]
              frame False {
              }
              frame True {
                n268 = Send Notification(notification=w649, notifier=w650) -> ()  [unwired: 1 in, 2 out]
              }
            }
          }
          frame "get_loop_conditional_terminal" {
            # "Returns the conditional terminal of a while- or for-loop (if enabled), to be used with connect_objects (as to_object_id, with index 0)."
            n269 = Variant To Data(error in=w661, type=T26 {"loop_id"=0, "Wait Notifier"=refnum, "wait for reply"=FALSE} ("get_loop_conditional_terminal Argument"), Variant=w658) -> (data=w652:T26, error out=w659:errorcluster)
            n270 = Unbundle By Name(w652) -> ("Wait Notifier"=w656:refnum<notifier>, "wait for reply"=w655:bool)  [unwired: 1 out]
            n271 = call "Do Get Cond Terminal.vi"("error in (no error)"=w659, "get_loop_conditional_terminal Argument"=w652, "Data Cluster in"=w660) -> ("error out"=w653:errorcluster, "get_loop_conditional_terminal (Reply Payload)"=w654:T57, "Data Cluster out"=w651:T2)  [unwired: 6 in]
            n272 = case "DQMH_FIRE_NOTIFIER" shown="True" w655 {
              tunnel: w656 -> [_ w663]
              tunnel: w654 -> [_ w662]
              frame False {
              }
              frame True {
                n273 = Send Notification(notification=w662, notifier=w663) -> ()  [unwired: 1 in, 2 out]
              }
            }
          }
          frame "show_conditional_terminal" {
            # "Shows or hides the conditional terminal of a for loop."
            n274 = Variant To Data(error in=w674, type=T27 {"loop_id"=0, "show"=FALSE, "Wait Notifier"=refnum, "wait for reply"=FALSE} ("show_conditional_terminal Argument"), Variant=w671) -> (data=w665:T27, error out=w672:errorcluster)
            n275 = Unbundle By Name(w665) -> ("Wait Notifier"=w669:refnum<notifier>, "wait for reply"=w668:bool)  [unwired: 2 out]
            n276 = call "do show conditional terminal.vi"("error in (no error)"=w672, "show_conditional_terminal Argument"=w665, "Data Cluster in"=w673) -> ("error out"=w666:errorcluster, "show_conditional_terminal (Reply Payload)"=w667:T58, "Data Cluster out"=w664:T2)  [unwired: 6 in]
            n277 = case "DQMH_FIRE_NOTIFIER" shown="True" w668 {
              tunnel: w669 -> [_ w676]
              tunnel: w667 -> [_ w675]
              frame False {
              }
              frame True {
                n278 = Send Notification(notification=w675, notifier=w676) -> ()  [unwired: 1 in, 2 out]
              }
            }
          }
          frame "get_loop_iteration_terminal" {
            # "Returns the loops iteration terminal to be used for wiring."
            n279 = Variant To Data(error in=w687, type=T28 {"loop_id"=0, "Wait Notifier"=refnum, "wait for reply"=FALSE} ("get_loop_iteration_terminal Argument"), Variant=w684) -> (data=w678:T28, error out=w685:errorcluster)
            n280 = Unbundle By Name(w678) -> ("Wait Notifier"=w682:refnum<notifier>, "wait for reply"=w681:bool)  [unwired: 1 out]
            n281 = call "do get loop iteration terminal.vi"("error in (no error)"=w685, "get_loop_iteration_terminal Argument"=w678, "Data Cluster in"=w686) -> ("error out"=w679:errorcluster, "get_loop_iteration_terminal (Reply Payload)"=w680:T59, "Data Cluster out"=w677:T2)  [unwired: 6 in]
            n282 = case "DQMH_FIRE_NOTIFIER" shown="True" w681 {
              tunnel: w682 -> [_ w689]
              tunnel: w680 -> [_ w688]
              frame False {
              }
              frame True {
                n283 = Send Notification(notification=w688, notifier=w689) -> ()  [unwired: 1 in, 2 out]
              }
            }
          }
          frame "Read Config Data" {
            # "Reads the config data from the config file."
            n284 = call <vilib>:"Application Directory.vi"() -> ("Application Directory"=w699:path)
            n285 = Strip Path(path=w699) -> (stripped path=w698:path)  [unwired: 1 out]
            n286 = Build Path(base path=w698, name or relative path="config.json") -> (appended path=w696:path)
            n287 = Unbundle By Name(w693) -> ("Config Data"=w692:T3)
            n288 = Read from Text File(file (use dialog)=w696, error in=w701) -> (text=w694:string, error out=w700:errorcluster)  [unwired: 2 in, 2 out]
            n289 = Unflatten From JSON(JSON string=w694, type and defaults=w692, error in (no error)=w700) -> (value=w690:T3, error out=w695:errorcluster)  [unwired: 4 in]
            n290 = Bundle By Name(cluster=w693, "Config Data"=w690) -> (w691:T2)
          }
          frame "get_allowed_paths" {
            # "Returns the Directories that the Server can write files/folders to. If you try to write to other locations you will receive an error. If asked to save to a relative path, use this function to build the full path."
            n291 = Variant To Data(error in=w713, type=T30 {"Wait Notifier"=refnum, "wait for reply"=FALSE} ("get_allowed_paths Argument"), Variant=w712) -> (data=w710:T30, error out=w702:errorcluster)
            n292 = Unbundle By Name(w705) -> ("Config Data.Allowed Paths"=w704:string[])
            n293 = Unbundle By Name(w710) -> ("Wait Notifier"=w709:refnum<notifier>, "wait for reply"=w708:bool)
            n294 = for {
              tunnel: w704 -> [w716] mode=indexing
              tunnel: [w714] -> w703 mode=concatenating
              n295 = Format Into String(format string="\"%s\", ", w716) -> (resulting string=w714:string)  [unwired: 2 in, 1 out]
            }
            n296 = Bundle By Name(cluster=T55 {"Allowed Paths"="", "error"={"status"=FALSE, "code"=0, "source"=""}} ("get_allowed_paths (Reply Payload)"), "Allowed Paths"=w703, "error"=w702) -> (w707:T55)
            n297 = case "DQMH_FIRE_NOTIFIER" shown="True" w708 {
              tunnel: w709 -> [_ w718]
              tunnel: w707 -> [_ w717]
              frame False {
              }
              frame True {
                n298 = Send Notification(notification=w717, notifier=w718) -> ()  [unwired: 1 in, 2 out]
              }
            }
          }
          frame "create_project" {
            # "Creates a new Project at the specified location"
            n299 = Variant To Data(error in=w729, type=T31 {"File Path"="", "Wait Notifier"=refnum, "wait for reply"=FALSE} ("create_project Argument"), Variant=w726) -> (data=w719:T31, error out=w727:errorcluster)
            n300 = Unbundle By Name(w719) -> ("Wait Notifier"=w724:refnum<notifier>, "wait for reply"=w723:bool)
            n301 = call "Do create project.vi"("error in (no error)"=w727, "create_project Argument"=w719, "Data Cluster in"=w728) -> ("error out"=w721:errorcluster, "create_project (Reply Payload)"=w722:T60, "Data Cluster out"=w720:T2)  [unwired: 6 in]
            n302 = case "DQMH_FIRE_NOTIFIER" shown="True" w723 {
              tunnel: w724 -> [_ w731]
              tunnel: w722 -> [_ w730]
              frame False {
              }
              frame True {
                n303 = Send Notification(notification=w730, notifier=w731) -> ()  [unwired: 1 in, 2 out]
              }
            }
          }
          frame "Set Working Directory" {
            # "Sets the allowed directory for the AI. This function shall not be exposed to the LLM."
            n304 = Variant To Data(error in=w740, type=T32 {"Working Directory Folder Path"=[]} ("Set Working Directory Argument"), Variant=w737) -> (data=w735:T32, error out=w738:errorcluster)
            n305 = Unbundle By Name(w735) -> ("Working Directory Folder Path"=w733:path[])
            n306 = Path To String(path=w733) -> (string=w732:string[])
            n307 = Bundle By Name(cluster=w739, "Config Data.Allowed Paths"=w732) -> (w734:T2)
          }
          frame "open_vi" {
            # "Opens a vi from inside the allowed paths and returns an id to further use it, similar to the new_vi tool."
            n308 = Variant To Data(error in=w751, type=T33 {"vi_path"="", "Wait Notifier"=refnum, "wait for reply"=FALSE} ("open_vi Argument"), Variant=w748) -> (data=w741:T33, error out=w749:errorcluster)
            n309 = Unbundle By Name(w741) -> ("Wait Notifier"=w746:refnum<notifier>, "wait for reply"=w745:bool)  [unwired: 1 out]
            n310 = call "Do Open Vi.vi"("error in (no error)"=w749, "open_vi Argument"=w741, "Data Cluster in"=w750) -> ("error out"=w743:errorcluster, "open_vi (Reply Payload)"=w744:T61, "Data Cluster out"=w742:T2)  [unwired: 6 in]
            n311 = case "DQMH_FIRE_NOTIFIER" shown="True" w745 {
              tunnel: w746 -> [_ w753]
              tunnel: w744 -> [_ w752]
              frame False {
              }
              frame True {
                n312 = Send Notification(notification=w752, notifier=w753) -> ()  [unwired: 1 in, 2 out]
              }
            }
          }
          frame "---Copy This Frame---" {
            # "Duplicate this frame when creating new messages.  Change this comment in the duplicated frame to describe this message."
            n313 = Merge Errors(w756) -> (w755:errorcluster)
          }
          frame "---Exit and Error Handling---" {
            # "Separator - The following cases handle errors and exit messages."
          }
          frame "Simulate MHL Error" {
            # "#DQMH_HowTo The 'Simulate MHL Error' button  illustrates how the MHL handles errors. This event is instructional in nature and can be removed."
            # "Simulate an error occurring at the MHL"
            n314 = call "Module Name--constant.vi"() -> ("Module Name"=w760:string)  [unwired: 11 in]
            n315 = Format Into String(format string="Simulated error originating at Message Handling Loop in %s", w760) -> (resulting string=w761:string)  [unwired: 2 in, 1 out]
            n316 = call <vilib>:"Error Cluster From Error Code.vi"("show call chain? (False)"=TRUE, "error message (\"\")"=w761, "error code (0)"=5001) -> ("error out"=w765:errorcluster)  [unwired: 6 in]
            n317 = Merge Errors(w767, w765) -> (w766:errorcluster)
          }
          frame "Error" {
            # "#DQMH_CodeRecommended - If the module is running in standalone mode (External Launch = FALSE), this code will pop up an error dialog and call the 'Exit' message if an error occurs. Add more fine-grained error management here."
            # "Error - Check the error message data and respond accordingly. This message is sent by the \"Error Handler\" VIs at the end of each loop in this application."
            n318 = property on="Property Node" class="Module Admin"(reference=w770) -> ("Accessors:External Launch"=w769:bool)  [unwired: 1 in, 2 out]
            n319 = Variant To Data(error in=w778, type=errorcluster {"status"=FALSE, "code"=0, "source"=""} ("error constant"), Variant=w772) -> (data=w768:errorcluster, error out=w776:errorcluster)
            n320 = local write "error out"(w768) -> ()
            n321 = call "Error Reported.vi"("Error"=w768) -> ()  [unwired: 10 in, 1 out]
            n322 = case shown="False" w769 {
              tunnel: [w783 _] -> w775
              tunnel: w771 -> [w781 _]
              tunnel: w768 -> [w782 _]
              frame False {
                n323 = disable-structure shown="Default" {
                  disable-tunnel: w782 -> [w784 _]
                  frame condition #0 (active) {
                    # "If the module is running standalone, then pop up an error dialog and call the \"Exit\" message."
                    n324 = call <vilib>:"Simple Error Handler.vi"("error in (no error)"=w784) -> ()  [unwired: 4 in, 5 out]
                  }
                  frame condition #1 {
                    # "To prevent the Simple Error Handler VI from being loaded (e.g. when deploying to a Real-Time target), add the Conditional Disable Symbol \"DQMH_Disable_SEH\" to your project and set it to TRUE."
                  }
                }
                n325 = call-poly <vilib>:"Delacor_lib_QMH_Enqueue Message (poly).vi"("Priority Message? (F)"=TRUE, "Message"="Exit", "Message Queue in"=w781) -> ("error out"=w783:errorcluster)  [unwired: 7 in, 1 out]
              }
              frame True {
                # "If the module was launched externally, calling the Error Reported broadcast VI is the only action performed by the \"Error\" message. The module's caller can then process the error appropriately."
              }
            }
            n326 = Merge Errors(w776, w775) -> (w774:errorcluster)
          }
          frame "Exit" {
            w789 = 91  # 91: not all Exit messages will have an argument
            w791 = TRUE  # Stop the VI
            # "Release the message queue reference"
            # "#DQMH_CodeNeeded - Add any required cleanup code here."
            # "Exit - Exit the application."
            n327 = Variant To Data(error in=w799, type=T5 {"Origin"="", "Exit via Stop Module Req?"=FALSE, "Wait for Module to stop?"=FALSE} ("Stop Argument"), Variant=w790) -> (data=w787:T5, error out=w796:errorcluster)
            n328 = call <vilib>:"Clear Errors.vi"("error in (no error)"=w796, "specific error code to clear (0: all)"=w789) -> ("error out"=w798:errorcluster)  [unwired: 4 in, 1 out]
            n329 = control-ref of="This VI"() -> (w786:refnum<vi>)
            n330 = call-dynamic "Delacor_lib_QMH_Release Message Queue.vi"("error in"=w798, "Message Queue"=w793) -> ("error out"=w797:errorcluster)  [unwired: 9 in]
            n331 = call "Handle Exit.vi"("Stop Argument"=w787, "Admin in"=w785, "VI reference"=w786) -> ("error out"=w795:errorcluster)  [unwired: 7 in, 1 out]
            n332 = Merge Errors(w797, w795) -> (w794:errorcluster)
            n333 = call "Error Reported.vi"("Error"=w794) -> ()  [unwired: 10 in, 1 out]
          }
          frame Default {
            # "'Default' case only runs if there is a message that isn't defined in any of the other cases.  Output a programming error."
            n334 = call "Module Name--constant.vi"() -> ("Module Name"=w804:string)  [unwired: 11 in]
            n335 = Format Into String(format string="The invalid message string \"%s\" was received in the Message Handling Loop for module \"%s\".", w805, w804) -> (resulting string=w800:string)  [unwired: 2 in, 1 out]
            n336 = call <vilib>:"Error Cluster From Error Code.vi"("show call chain? (False)"=TRUE, "error message (\"\")"=w800, "error code (0)"=1) -> ("error out"=w807:errorcluster)  [unwired: 6 in]
            n337 = Merge Errors(w808, w807) -> (w809:errorcluster)
          }
        }
        n338 = call-dynamic "Delacor_lib_QMH_Error Handler - Message Handling Loop.vi"("error in"=w325, "Message Queue in"=w324) -> ("dup error in"=w326:errorcluster)  [unwired: 8 in, 1 out]
      }
    }
    frame Error {
      # "Synchronize Caller Events.vi will inform Start Module.vi that the module has launched and will let the code calling Start Module.vi register for broadcasts and would permit the caller receive the broadcast that an error occurred at launch time."
      n339 = call-dynamic "Delacor_lib_QMH_Release Message Queue.vi"("error in"=w817, "Message Queue"=w810) -> ("error out"=w816:errorcluster)  [unwired: 9 in]
      n340 = call "Synchronize Caller Events.vi"("Singleton Module Admin in"=w811) -> ("error out"=w818:errorcluster)  [unwired: 9 in, 1 out]
      n341 = call "Module Name--constant.vi"() -> ("Module Name"=w814:string)  [unwired: 11 in]
      n342 = Format Into String(format string="An error occurred during initialization. %s is no longer running.", w814) -> (resulting string=w812:string)  [unwired: 2 in, 1 out]
      n343 = Merge Errors(w816, w818) -> (w819:errorcluster)
      n344 = call "Error Reported.vi"("Additional Information"=w812, "Error"=w819) -> ()  [unwired: 9 in, 1 out]
    }
  }
  n345 = Merge Errors(w14, w17) -> (w13:errorcluster)
  n346 = call "Close Module.vi"("error in"=w13, "Module Admin in"=w8) -> ("error out"=w15:errorcluster, "External Launch"=w1:bool, "Module Admin out"=w2:refnum<class "Delacor_lib_QMH_Module Admin.lvclass">)  [unwired: 7 in]
  n347 = Unregister For Events(event registration refnum=w7, error in=w15) -> (error out=w12:errorcluster)
  "error out" <- w12
  n348 = case "External Launch?" shown="True" w1 {
    tunnel: w12 -> [_ w820]
    frame False {
    }
    frame True {
      n349 = case shown="No Error" w820 {
        frame No Error {
          n350 = invoke on="Invoke Node" class="VI" method="FP.Close"() -> ()  [unwired: 3 in, 3 out]
        }
        frame Error {
          n351 = disable-structure shown="Default" {
            frame condition #0 (active) {
              n352 = invoke class="VI" method="FP.Open"("Activate"=TRUE ("Activate?")) -> ()  [unwired: 4 in, 5 out]
            }
            frame condition #1 {
              # "Don't show panel on error if running inside a built EXE."
            }
          }
        }
      }
    }
  }
  n353 = local write "Module Admin"(w2) -> ()
